vi "GUI_Bella_Control_Center_Staging.vi"() -> ()   [LabVIEW 2020]
uses:
  Shared/GUI_Template/GUI_master/tcp_new_data_event.ctl
  Shared/GUI_Template/GUI_master/tcp new data cluster.ctl
  GUI_TestStand/Fire button.ctl
  Device Drivers/DG645/subVIs/TriggerSource_TypDef.ctl
  delay scan start and end.ctl
  <vilib>/Utility/config.llb/Write Key (I32).vi
  <vilib>/Platform/browser.llb/Open URL in Default Browser (string).vi
  <vilib>/Utility/config.llb/NI_LVConfig.lvlib
panel:
  in  "GUIdevice 33":string="FLIP-1BL-Tel4FoilND1"
  in  "Position::33":enum16{"Unknown", "Position1", "Position2"}(ring) caption="1BLTel4Foil"
  in  "Uniblitz":bool=TRUE
  in  "value13::42":dbl=0.006 caption="Jet SC ChF PostScan" min=-9999999.0 max=9999999.0 format="%#_3f"
  in  "value12::42":dbl=0.006 caption="Jet  SC ChF Scan" min=-9999999.0 max=9999999.0 format="%#_3f"
  in  "GUIdevice 42":string="MANPAR-BELLA-OFI"
  in  "value15::42":dbl=0.006 caption="SC ChA PostScan" min=-9999999.0 max=9999999.0 format="%#_3f"
  in  "value14::42":dbl=0.006 caption="SC ChA Scan" min=-9999999.0 max=9999999.0 format="%#_3f"
  out "density down (10^18/cc)":dbl
  out "density up (10^18/cc)":dbl
  in  "Amplitude.Ch AB::13":dbl caption="Cap Trigger (V)" min=0.5 max=5.0 format="%.3p"
  in  "Delay.Ch A::13":dbl caption="Discharge delay A" min=-0.9 max=0.9 format="%.3p"
  in  "GUIdevice 13":string="DDG-AA-SRS2"
  in  "pressure::29":dbl caption="Dopant P set (Torr)" min=0.0 max=500.0 format="%.2f"
  out "pressure2::19":dbl caption="Pressure act DS (Torr)" min=-100.0 max=500.0 format="%.2f"
  out "pressure::19":dbl caption="Stage1 P act US (Torr)" min=-100.0 max=500.0 format="%.2f"
  in  "Delay.Ch B::13":dbl caption="Cap Trigger width" min=0.0 max=1e-05 step=1e-05 format="%.3p"
  in  "pressure::26":dbl caption="APL Pressure (Torr)" min=0.0 max=50.0 format="%.2f"
  out "Data.Channel 2::14":dbl caption="Flow US (sccm)" min=0.0 max=1000.0 format="%.1f"
  in  "Data.Channel 2::11":dbl caption="Stage1 P set US (Torr)" min=0.0 max=1000.0 format="%.2f"
  in  "SlaveValue::11":dbl caption="Slave Value (%)" min=0.0 max=1000.0 format="%.1f"
  out "Data.Channel 1::14":dbl caption="Flow DS (sccm)" min=0.0 max=1000.0 format="%.1f"
  in  "Data.Channel 1::11":dbl caption="Stage1 P set DS (Torr)" min=0.0 max=1000.0 format="%.2f"
  in  "GUIdevice 19":string="GAUGE-PL1-CapPressure"
  in  "Position.Ch3::18":dbl caption="stage 2 longitudinal" min=0.0 max=78.0
  in  "Position.Ch2::18":dbl caption="Stage 2 transverse" min=-100.0 max=100.0
  in  "Position.Ch4::18":dbl caption="Stage 2 vertical" min=0.0 max=40.0
  in  "GUIdevice 18":string="STAGE-PL1-Zaber"
  in  "position::16":dbl caption="tape vertical (mm)" min=-48.0 max=0.0
  in  "hex pos for SMF focal scan":dbl=6.5 caption="hex pos for SMF focus" format="%#_13g"
  in  "dist SMF to cap entrance":dbl=6.5 caption="dist SMF to cap entrance\n+ve SMF upstream" format="%#_13g"
  in  "value11::42":dbl caption="SMF focus on HPD" min=-9999999.0 max=9999999.0
  out "Focus into cap":dbl
  in  "GUIdevice 16":string="STAGE-PL1-Vertical"
  in  "wangle::30":dbl caption="w" min=-10.0 max=10.0 step=0.01 format="%.5f"
  in  "vangle::30":dbl caption="v" min=-5.0 max=5.0 step=0.01 format="%.5f"
  in  "uangle::30":dbl caption="u" min=-5.0 max=5.0 step=0.01 format="%.5f"
  in  "ypos::30":dbl caption="y" min=-10.0 max=10.0 step=0.01 format="%.5f"
  in  "zpos::30":dbl caption="z" min=-10.0 max=10.0 step=0.01 format="%.5f"
  in  "xpos::30":dbl caption="x" min=-25.0 max=25.0 step=0.01 format="%.5f"
  in  "GUIdevice 30":string="HEX-PL1-3"
  in  "GUIdevice 29":string="PRC-PL1-Stage1-Dopant"
  in  "Position.Ch1::44":dbl caption="Current Position" min=0.0 max=150.0 format="%.3f"
  in  "Position.Channel 2::31":T1(ring) caption="Little Rick"
  in  "GUIdevice 27":string="DDG-AA-SRS3"
  in  "GUIdevice 26":string="PRC-PL1-PressureAPL"
  in  "GUIdevice 20":string="HV-PL1-Glassman"
  in  "GUIdevice 14":string="GAUGE-PL1-FlowStage1"
  in  "GUIdevice 11":string="PRC-PL1-Stage1"
  in  "amplitude.Channel_A::27":dbl caption="Caps Trig (V) c unpl?" min=-3.0 max=4.0 format="%.2f"
  in  "voltage::20":dbl caption="Discharge HV (kV)" min=0.0 max=40.0 format="%.2f"
  in  "Delay.Ch B::10":dbl=-1.631e-06 caption="UniblitzOpenTime B\n(0 closed, 0.07 default)" min=-0.1 max=15.0 format="%.4f"
  in  "value6::42":dbl=0.006 caption="PostScanRate ChF" min=0.1 max=1.0 format="%#_3f"
  in  "value1::43":bool=TRUE caption="GasJetOn"
  in  "value0::43":bool=TRUE caption="SCS"
  in  "Delay.Ch H::32":dbl caption="Time width H" min=-0.1 max=0.01 format="%.3p"
  in  "Delay.Ch G::32":dbl caption="jet open G" min=-0.1 max=0.1 format="%.3p"
  in  "Delay.Ch D::32":dbl caption="Time Width D" min=-0.1 max=0.01 format="%.3p"
  in  "Delay.Ch E::32":dbl caption="jet open E" min=-0.1 max=0.03 format="%.3p"
  in  "Delay.Ch F::32":dbl caption="Time width F" min=-0.1 max=0.01 format="%.3p"
  in  "Delay.Ch C::32":dbl caption="jet open C" min=-0.1 max=0.1 format="%.3p"
  out "got manpar ofi bool data":bool
  out "got manpar ofi data":bool
  out "set expt editor":bool
  in  "Delay.Ch F::10":dbl=-1.631e-06 caption="Delay F" min=-0.1 max=10.0 format="%.4f"
  in  "Amplitude.Ch GH::10":dbl=-1.631e-06 caption="Shot Shutter V" min=0.5 max=5.0 format="%.1f"
  in  "Rate (Hz)":dbl=0.3
  in  "Allow Fire Continues":bool
  out "Fire continues Indicator":bool caption="firing"
  in  "Fire Button":T2=TRUE
  in  "Trigger.Source::10":T3 caption="SRS Trigger Mode"
  in  "value5::42":dbl=0.006 caption="1BL-2BL-\nSplitter-Rpcnt" min=-9999999.0 max=9999999.0 format="%#_6p"
  in  "value6::43":bool=TRUE caption="GhostFoil-In"
  in  "value5::43":bool=TRUE caption="1BL-Energy\nMeter-In"
  in  "value4::43":bool=TRUE caption="2BLFoil-In"
  in  "value3::43":bool=TRUE caption="1BLFoil-In"
  in  "value2::43":bool=TRUE caption="ClunkerIn"
  out "CurrentStatus":string
  in  "MoveStage":bool
  in  "GUIdevice 44":string="STAGE-LT-Megattenuator"
  in  "GUIdevice 43":string="MANPAR-BELLA-OFI-Boolean"
  in  "Pressure.device 2::39":dbl caption="Dopant pressure\nLow1down" min=-20.0 max=500.0 format="%.3f"
  out "HPD2 to match HPD":dbl
  out "HPD - focus":dbl
  in  "value1::42":dbl=230.0 caption="1BL focus pos" min=-9999999.0 max=9999999.0
  in  "position::23":dbl caption="position HPD2" min=0.0 max=600.0 format="%.1f"
  in  "position::3":dbl caption="position HPD" min=0.0 max=600.0 format="%.1f"
  in  "Save \ncreenshots":bool
  out "error out":errorcluster
  out "Hpd pos for jet exit":dbl
  in  "value2::42":dbl=276.0 caption="jet exit on hpd for hexX=0" min=-9999999.0 max=9999999.0
  in  "GUIdevice 41":string="STAGE-PL1-JetLength"
  in  "position::41":dbl caption="Jet Length pos" min=0.0 max=50.0 format="%.1f"
  out "lp mode HPDplane\n - HPD ref pos":dbl
  out "height above jet":dbl
  in  "value3::42":dbl=2.6 caption="zpos for 0 above jet" min=-9999999.0 max=9999999.0
  out "1BL delay (ns)\n+ is 1BL after 2BL":dbl
  in  "Position.Axis 1::8":dbl caption="1BL delay (mm)" min=-500.0 max=500.0 format="%.1f"
  in  "GUIdevice 8":string="STAGE-LT-1BLDelay"
  in  "Position.Channel 5::25":dbl caption="SMFiber (45in, 1out)" min=-60.0 max=55.0 format="%.1f"
  in  "Thales.DIAG_CU_Output_Percent_1::37":dbl caption="Amp2 att (%)" min=1.0 max=100.0 step=500.0 format="%.2f"
  in  "GUIdevice 37":string="SVE-LT-Thales"
  in  "Pressure.device 1::39":dbl caption="Hydrogen pressure\nHigh500" min=15.0 max=500.0 format="%.3f"
  in  "GUIdevice 39":string="PRC-PL1-HighPressure"
  in  "Scan":T4(ring)
  in  "LogTable":bool
  in  "New Google\nExpLog for new day?":bool=TRUE
  out "standard output":string
  in  "Create Log":bool caption="LogTable"
  in  "GUIdevice 38":string="STAGE-2BL-Compressor"
  in  "Position.Axis 1::38":dbl caption="Comp2 Translation" min=0.0 max=20.0 format="%.3f"
  in  "Position.Channel 5::31":T1(ring) caption="FROG foil"
  in  "AnalogOutput.Channel 1::36":dbl caption="M4A att (V)" min=0.0 max=5.0 step=500.0 format="%.2f"
  in  "GUIdevice 36":string="ATT-2BL-M4A"
  in  "GUIdevice 35":string="ATT-2BL-DM"
  in  "AnalogOutput.Channel 1::35":dbl caption="2BL DM att (V)" min=0.0 max=5.0 step=500.0 format="%.2f"
  in  "Delay.Ch B::32":dbl caption="Time width B" min=-0.1 max=0.01 format="%.3p"
  in  "Delay.Ch A::32":dbl caption="jet open A" min=-0.1 max=0.1 format="%.3p"
  in  "GUIdevice 32":string="DDG-AA-SRSGasJet-645"
  in  "position::6":dbl caption="LPmode stage long (605 safe)" min=0.0 max=50.0 format="%.1f"
  in  "GUIdevice 6":string="STAGE-PL1-LPmodeLong"
  in  "EnableMotor::6":bool caption="LPmode motor \nstatus"
  in  "GUIdevice 4":string="STAGE-PL1-Capstage1"
  in  "GUIdevice 31":string="FLIP-AA-1Wire"
  out "Crystal2":enum16{"In", "Out", "Unknown"}(ring)
  in  "wangle::28":dbl caption="w" min=-2.0 max=2.0 step=0.01 format="%.5f"
  in  "vangle::28":dbl caption="v" min=-5.0 max=5.0 step=0.01 format="%.5f"
  in  "uangle::28":dbl caption="u" min=-1.0 max=1.0 step=0.01 format="%.5f"
  in  "ypos::28":dbl caption="y" min=-3.0 max=3.0 step=0.01 format="%.5f"
  in  "zpos::28":dbl caption="z" min=-12.5 max=12.5 step=0.01 format="%.5f"
  in  "xpos::28":dbl caption="x" min=-10.0 max=15.0 step=0.01 format="%.5f"
  in  "GUIdevice 28":string="HEX-PL1-2"
  in  "Position.Channel 1::25":dbl caption="LPmode kicker (~1in, 75out)" min=-75.0 max=79.0 format="%.1f"
  in  "GUIdevice 25":string="STAGE-PL1-Smaract"
  in  "Heater Alignment Directions":bool
  in  "Position.Axis 3::15":dbl caption="XY" min=-3.0 max=16.0 format="%.4f"
  in  "Position.Axis 2::15":dbl caption="Y" min=-3.0 max=17.0 format="%.4f"
  in  "Position.Axis 1::15":dbl caption="X" min=-3.0 max=13.0 format="%.4f"
  in  "GUIdevice 24":string="STAGE-HEAT-TL1"
  in  "GUIdevice 23":string="STAGE-HPD-Far"
  in  "GUIdevice 22":string="MANPAR-BELLA-FireCont"
  out "Absolute discharge timing":dbl caption="delay from pk" format="%#.3p"
  in  "value0::22":bool caption="Fire continuosly"
  in  "GUIdevice 15":string="MCD-HEAT-ESP1"
  in  "GUIdevice 17":string="DDG-AA-SRS0"
  out "error IO 2":errorcluster
  out "fire::10":string
  out "tcp data event":T5
  in  "UDP error message":string
  in  "GUIdevice 2":string="MANPAR-BELLA-General"
  in  "GUIdevice 10":string="DDG-AA-ShotCntrl"
  in  "GUIdevice 1":string="HEX-PL1-1"
  in  "GUIdevice 3":string="STAGE-HPD-Tel"
  in  "<command>::1":bool caption="ABORT\nHEXAPOD"
  in  "Step size":dbl min=-22.0 max=22.0 format="%.5f"
  in  "wangle::1":dbl caption="w (F11 F12)" min=-6.0 max=6.0 step=0.01 format="%.5f"
  in  "vangle::1":dbl caption="v (F9 F10)" min=-6.0 max=1.0 step=0.01 format="%.5f"
  in  "uangle::1":dbl caption="u (F7 F8)" min=-6.0 max=6.0 step=0.01 format="%.5f"
  in  "ypos::1":dbl caption="y (F3 F4)" min=-8.0 max=8.0 step=0.01 format="%.5f"
  in  "zpos::1":dbl caption="z (PgU PgD)" min=-12.0 max=15.0 step=0.01 format="%.5f"
  in  "xpos::1":dbl caption="x (F1 F2)" min=-25.0 max=25.0 step=0.01 format="%.5f"
  in  "Position.Axis 1::9":dbl caption="Comp1 Translation" min=-50.0 max=50.0 format="%.3f"
  in  "GUIdevice 9":string="STAGE-1BL-Compression"
  in  "stop":bool
  # "Jet"
  # "BELLA CONTROL CENTER"
  # "Manual Pars"
  # "Scan"
  # "CAP"
  # "Tape Hex (sm)"
  # "1wire"
  # "needs manpar-bella-ofi on\nMANPAR-BELLA-OFI-Boolean"
  # "Discharge timing (s)"
  # "off overrides \nto 0 ->"
  # "Heater timing (s)"
  # "Attenuate"
  # "Megattenuator Stage"
  # "IN"
  # "OUT"
  # "HEX 2 APL"
  # "DG"
  # "Compressors"
  # "AB Uniblitz\nCD AND gate SRS2\nEF trigs SRS4 (jet)\nGH big SCS"
  # "Note: APL actually R660um and L 13cm"
  # "pos1=in"
  # "Heater Alignment"
  # "Heat ESP0"
  # "Heat ESP1"
  # "Heat Pico"
  # "HPD Stage"
  # "HEX 1 cap"
  # "\"+x\" is laser propagation direction"
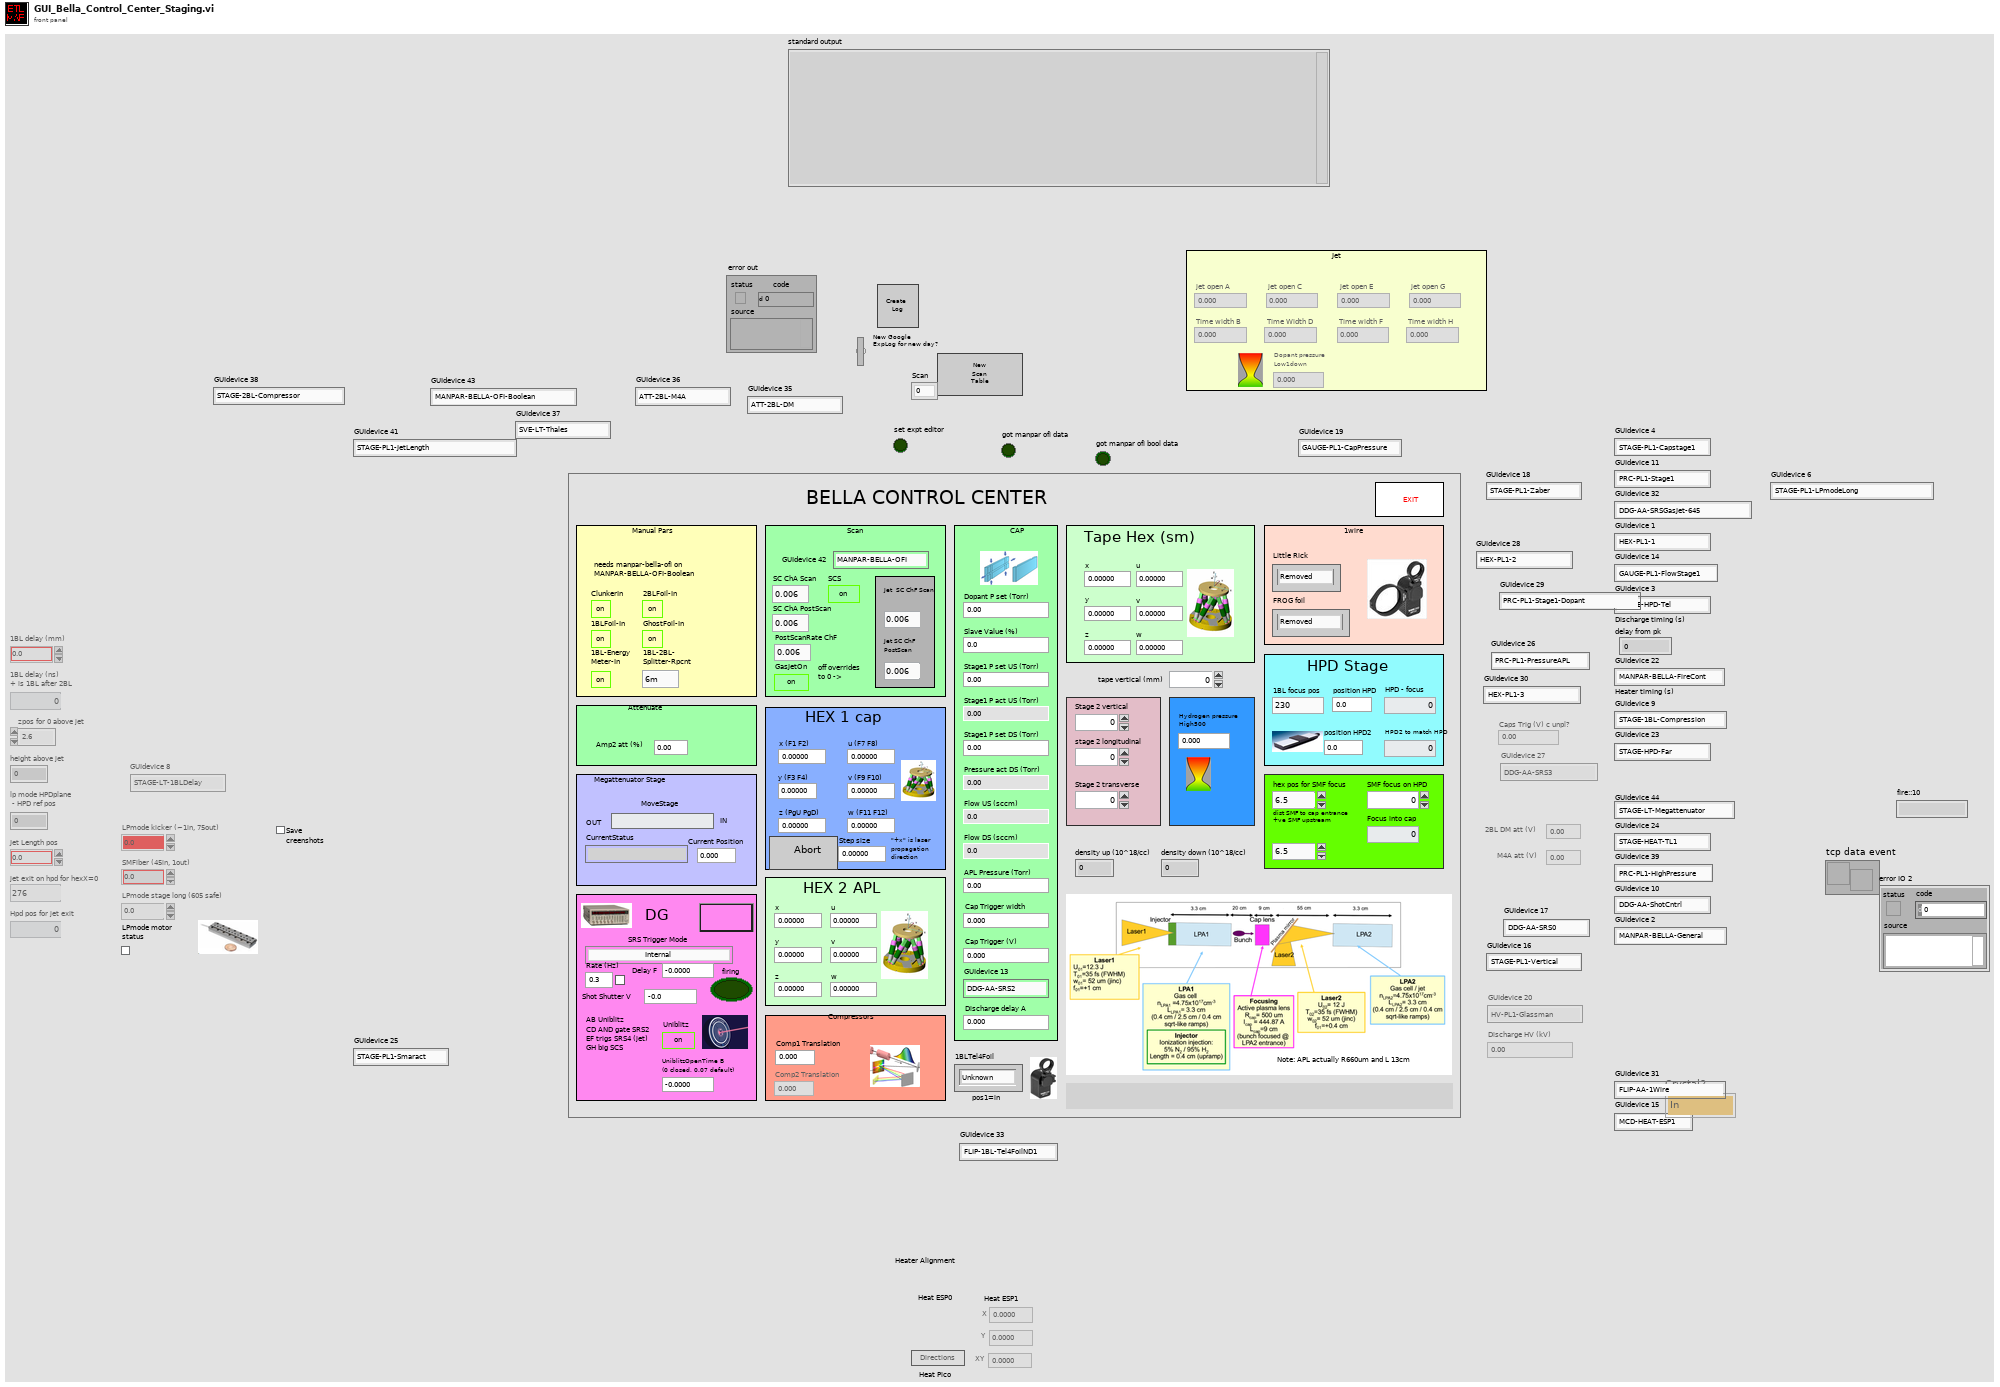
[diagram p1: front panel]
types:
  T1 = enum16{"Removed", "Inserted", "Unknown", "Moving"}
  T2 = typedef "Fire button.ctl" = bool
  T3 = typedef "TriggerSource_TypDef.ctl" = enum16{"Internal", "External rising edges", "External falling edges", "Single shot external rising edges", "Single shot external falling edges", "Single shot", "Line"}
  T4 = enum16{"0", "1", "2", "3", "4", "5", "6", "7", "8", "9", "10", "11", "12", "13", "14", "15", "16", "17", "18", "19", "20", "21", "22", "23", "24", "25", "26", "27", "28", "29", "30", "31", "32", "33", "34", "35", "36", "37", "38", "39", "40", "41", "42", "43", "44", "45", "46", "47", "48", "49", "50", "51", "52", "53", "54", "55", "56", "57", "58", "59", "60", "61", "62", "63", "64", "65", "66", "67", "68", "69", "70", "71", "72", "73", "74", "75", "76", "77", "78", "79", "81", "82", "83", "84", "85", "86", "87", "88", "89", "90", "91", "92", "93", "94", "95", "96", "97", "98", "99", ""}
  T5 = typedef "tcp_new_data_event.ctl" = refnum<user-event>
  T6 = typedef "tcp new data cluster.ctl" = cluster{"EventEnum":enum16{"new data", "connection status update"}, "Device name":string}
  T7 = enum8{"Enabled", "Disabled", "Disabled and Grayed Out"}
  T8 = enum32{"invalid app kind", "Development System", "Run Time System", "Student Edition", "Embedded LabVIEW", "Evaluation", "Custom"}
  T9 = enum32{"Invalid", "Standard", "Closed", "Hidden", "Minimized", "Maximized"}
  T10 = typedef "delay scan start and end.ctl" = cluster{"Channel":string, "Scan Start":dbl, "Scan End":dbl}
  T11 = typedef "imagedata.ctl" = cluster{"image type":i32, "image depth":i32, "image":u8[], "mask":u8[], "colors":u32[], "Rectangle":cluster{"left":i16, "top":i16, "right":i16, "bottom":i16}}
  T12 = typedef "NI_LVConfig.lvlib/Config Data RefNum.ctl" = refnum<k1>
  T13 = cluster{"Core":cluster{"Current VI Reference":refnum<vi>, "Close Panel on Exit?":bool}, "Heater timing offset":dbl, "Discharge timing offset":dbl, "Jet trigger":bool, "Tik1":u32, "Tik2":u32, "Fire Continues Allowed":bool}
  T14 = cluster{"Current VI Reference":refnum<vi>, "Close Panel on Exit?":bool}
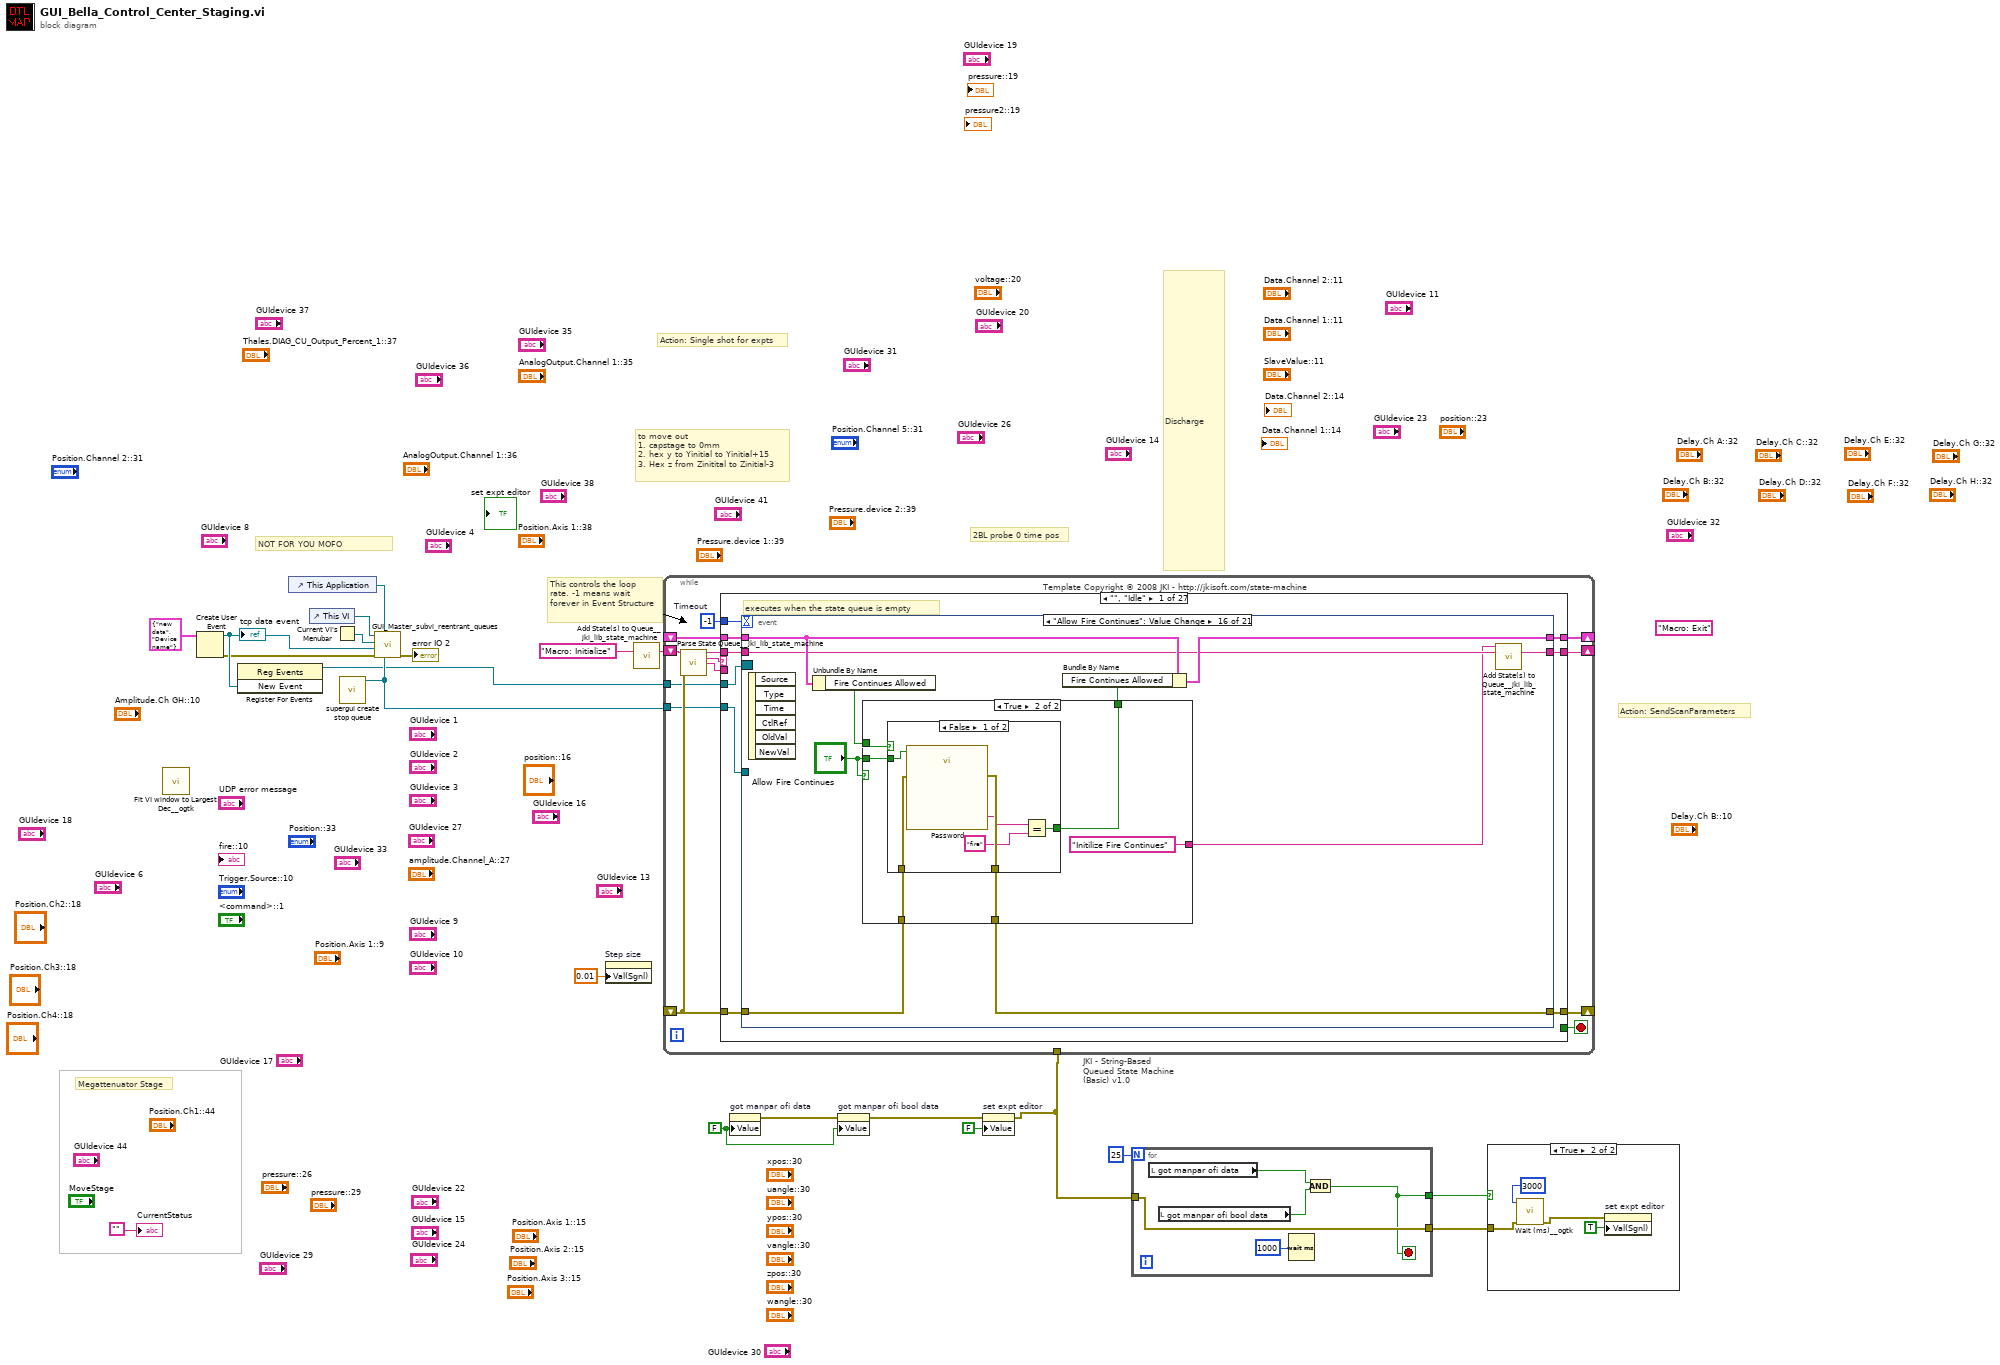
[diagram p0: block diagram]
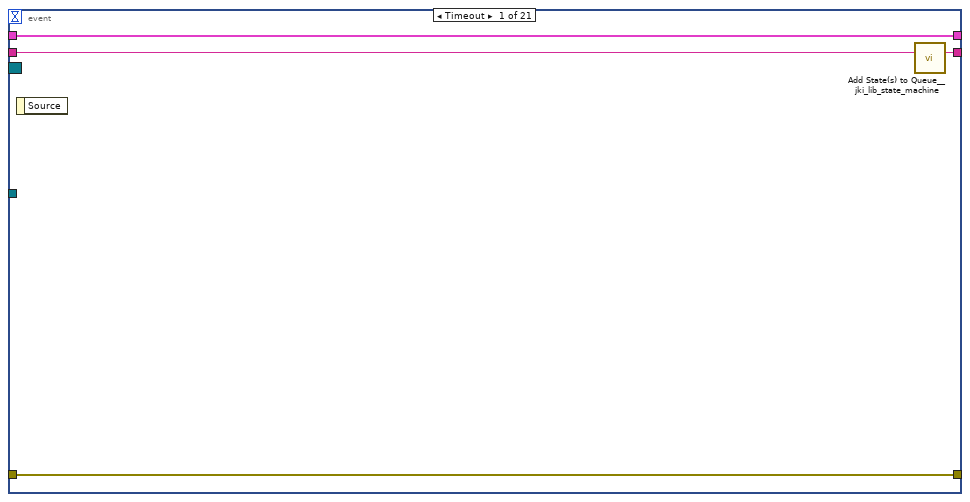
[diagram p3: hidden frame]
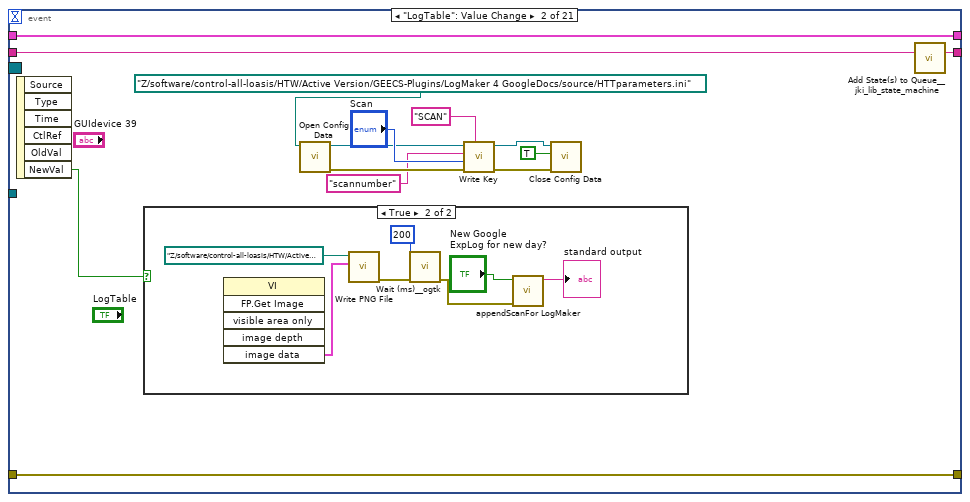
[diagram p4: hidden frame]
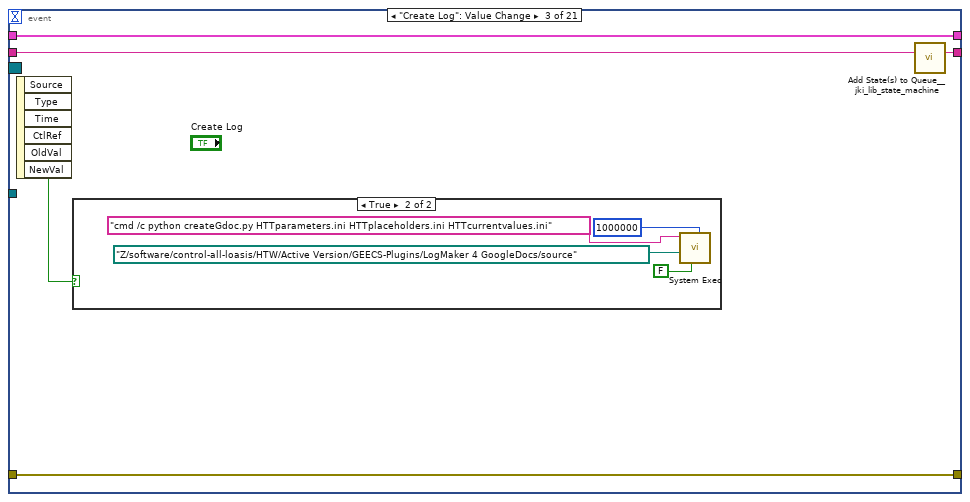
[diagram p6: hidden frame]
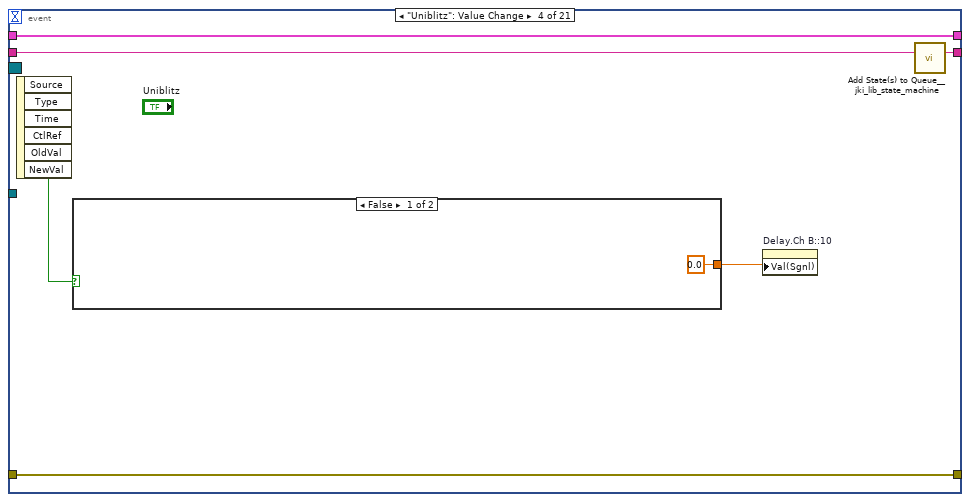
[diagram p8: hidden frame]
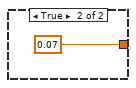
[diagram p9: hidden frame]
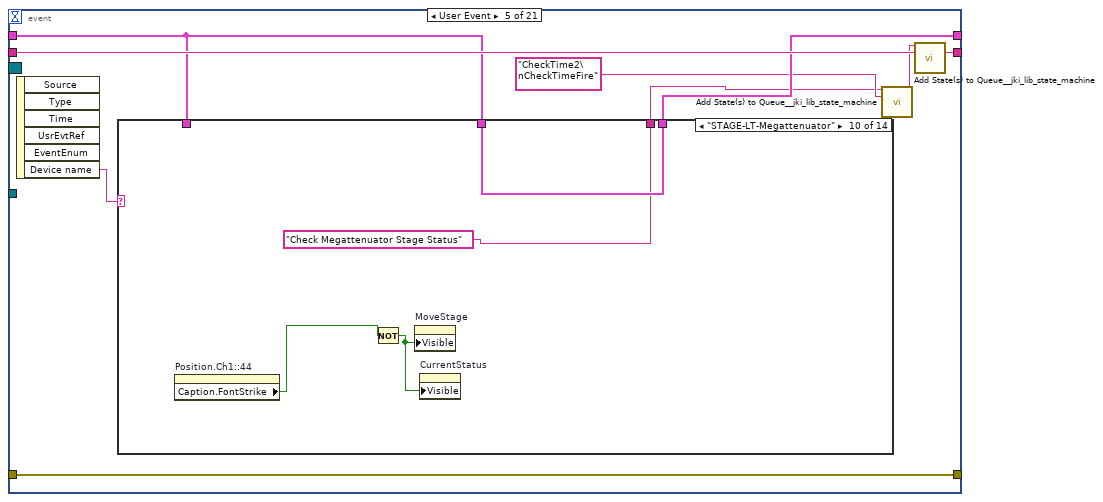
[diagram p10: hidden frame]
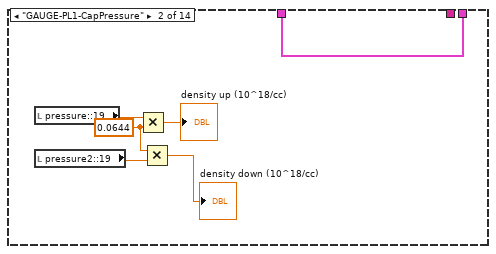
[diagram p12: hidden frame]
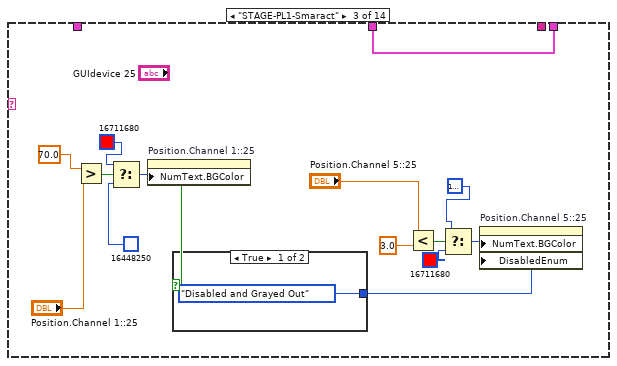
[diagram p13: hidden frame]
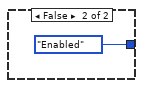
[diagram p14: hidden frame]
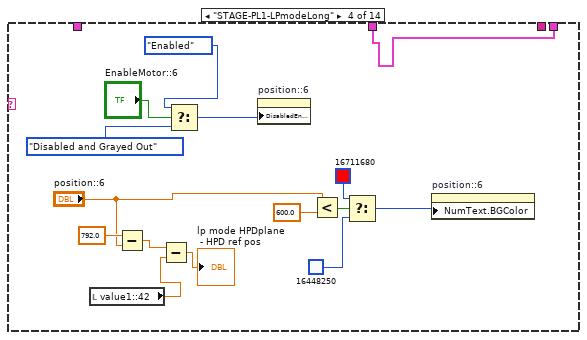
[diagram p15: hidden frame]
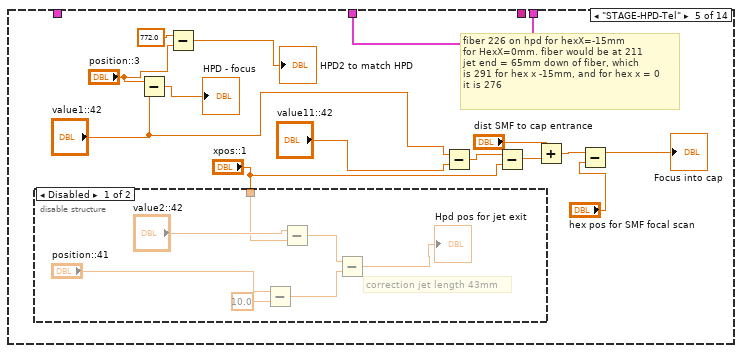
[diagram p16: hidden frame]
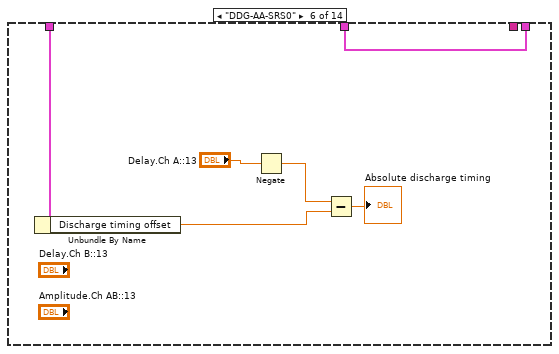
[diagram p18: hidden frame]
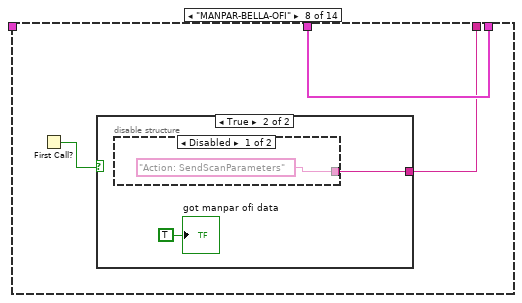
[diagram p20: hidden frame]
diagram:
  w5 = FALSE ("got manpar ofi data")
  (unwired) "Macro: Exit"
  # "Action: SendScanParameters"
  # "Discharge"
  # "Megattenuator Stage"
  # "2BL probe 0 time pos"
  # "Action: Single shot for expts"
  # "to move out\n1. capstage to 0mm\n2. hex y to Yinitial to Yinitial+15\n3. Hex z from Zinitital to Zinitial-3"
  # "This controls the loop rate. -1 means wait forever in Event Structure"
  # "NOT FOR YOU MOFO"
  n1 = call <userlib>:"Fit VI window to Largest Dec__ogtk.vi"() -> ()  [unwired: 6 in, 2 out]
  n2 = Create User Event(user event datatype=T6 {"EventEnum"=enum."new data", "Device name"="Device name"} ("New Event")) -> (user event=w20:refnum<user-event>, error out=w19:errorcluster)  [unwired: 1 in]
  "tcp data event" <- w20
  n3 = register-events(w20) -> (reference out=w10:refnum<event-registration>)  [unwired: 2 in, 1 out]
  n4 = control-ref of="This Application"() -> (w21:refnum<vi>)
  n5 = control-ref of="This VI"() -> (w14:refnum<vi>)
  n6 = Current VI's Menubar() -> (w17:refnum<k9>)
  n7 = call "supergui create stop queue.vi"() -> ("STOP Queue out"=w11:refnum<queue>)  [unwired: 11 in]
  n8 = call "GUI_Master_subvi_reentrant_queues.vi"("STOP Queue in"=w11, "This Application"=w21, "error in (no error)"=w19, "tcp data event"=w20, "Caller menu reference"=w17, "Caller VI ref"=w14) -> ("error out"=→"error IO 2":errorcluster)  [unwired: 5 in]
  n9 = property on="Step size" class="DigNum (strict)"("Val(Sgnl)"=0.01 ("Value (Signaling)")) -> ()  [unwired: 2 in, 2 out]
  n10 = call <vilib>:"Add State(s) to Queue__jki_lib_state_machine.vi"("State(s) in (\"\")"="Macro: Initialize") -> ("States Out"=w12:string)  [unwired: 14 in]
  n11 = property on="got manpar ofi data" class="Bool (strict)"("Value"=w5) -> (error out=w6:errorcluster)  [unwired: 2 in, 1 out]
  n12 = property on="got manpar ofi bool data" class="Bool (strict)"(error in=w6, "Value"=w5) -> (error out=w7:errorcluster)  [unwired: 1 in, 1 out]
  n13 = property on="set expt editor" class="Bool (strict)"(error in=w7, "Value"=FALSE ("set expt editor")) -> (error out=w4:errorcluster)  [unwired: 1 in, 1 out]
  n14 = while "JKI - String-Based Queued State Machine (Basic) v1.0" {
    shift-right: [w27] -> _
    shift-left: _ -> [w26]
    shift-right: [w30] -> _
    shift-left: _ -> [w24]
    shift-right: [w29] -> _
    shift-left: w12 -> [w31]
    tunnel: w10 -> [w23]
    tunnel: w11 -> [w22]
    tunnel: w4 -> [_]
    stop <- w28 stop-if-true
    w25 = -1  # Timeout
    # "Template Copyright © 2008 JKI - http://jkisoft.com/state-machine"
    n15 = call <vilib>:"Parse State Queue__jki_lib_state_machine.vi"("State Queue"=w31, "Error In (no error)"=w24) -> ("Remaining States"=w33:string, "Current State"=w34:string, "Arguments"=w32:string)  [unwired: 11 in]
    n16 = case shown="\"\", \"Idle\"" w34 {
      selector: w34 -> [_ _ w372 _ _ _ _ _ _ _ _ _ _ _ _ _ _ _ _ _ _ _ _ _ _ _ _]
      tunnel: w33 -> [w43 w371 w376 w394 w400 w405 w409 w420 w426 w430 w434 w440 w451 w477 w482 w495 w499 w505 w514 w551 w562 w574 w586 w595 w599 w634 w649]
      tunnel: w32 -> [_ _ _ _ _ _ _ _ _ _ _ w435 w445 _ _ _ _ _ _ _ _ _ _ _ _ _ _]
      tunnel: w26 -> [w41 w368 w374 w385 w397 w403 w406 _ w421 w427 w432 w438 w447 w474 w479 w492 w496 w502 w511 w539 w558 w568 w583 w593 w596 w631 w646]
      tunnel: [w40 w369 w378 w391 errorcluster {"status"=FALSE, "code"=0, "source"=""} ("error out") w402 w407 w417 w422 w428 w431 w436 w448 w475 w480 w493 w497 w503 w512 w549 w556 w563 w584 w590 w597 w632 w647] -> w30
      tunnel: w24 -> [w39 w369 w377 w391 w396 w402 w407 w417 w423 w428 w431 w437 w449 w475 w480 w493 w497 w503 w512 w549 w560 w564 w584 w591 w597 w632 w647]
      tunnel: [w42 w370 w375 w393 w399 w404 w408 w419 w425 w429 w433 w439 w450 w476 w481 w494 w498 w504 w513 w550 w561 w573 w585 w594 w598 w633 w648] -> w29
      tunnel: [_ _ _ _ _ TRUE _ _ _ _ _ _ _ _ _ _ _ _ _ _ _ _ _ _ _ _ _] -> w28
      tunnel: [w35 w368 w374 w392 w397 w403 w406 w418 w421 w427 w432 w438 w447 w474 w479 w492 w496 w502 w511 w548 w558 w567 w582 w593 w596 w631 w646] -> w27
      tunnel: w25 -> [w38 _ _ _ _ _ _ _ _ _ _ _ _ _ _ _ _ _ _ _ _ _ _ _ _ _ _]
      tunnel: w23 -> [w37 _ _ _ _ _ _ _ _ _ _ _ _ _ _ _ _ _ _ _ _ _ _ _ _ _ _]
      tunnel: w22 -> [w36 _ _ _ _ _ _ _ _ _ _ _ _ _ _ w484 _ _ _ _ _ _ _ _ _ _ _]
      frame "", "Idle" {
        # "executes when the state queue is empty"
        n17 = event shown="[15] \"Allow Fire Continues\": Value Change" {
          selector: w37 -> [_ _ _ _ _ _ _ _ _ _ _ _ _ _ _ _ _ _ _ _ _]
          dyn-events: _ -> [_ _ _ _ _ _ _ _ _ _ _ _ _ _ _ _ _ _ _ _ _]
          timeout: w38 -> [_ _ _ _ _ _ _ _ _ _ _ _ _ _ _ _ _ _ _ _ _]
          tunnel: w43 -> [w47 w61 w73 w83 w94 w215 w217 w222 w232 w242 w252 w262 w272 w278 w296 w305 w328 w333 w339 w341 w367]
          tunnel: [w46 w60 w72 w82 w93 w214 w218 w223 w233 w243 w253 w263 w273 w279 w296 w304 w328 w331 w339 w340 w366] -> w42
          tunnel: w41 -> [w44 w58 w70 w80 w90 w212 w220 w225 w235 w245 w255 w265 w275 w281 w295 w307 w329 w335 w338 w348 w364]
          tunnel: [w45 w59 w71 w81 w92 w213 w219 w224 w234 w244 w254 w264 w274 w280 w293 w310 w327 w334 w337 w347 w365] -> w40
          tunnel: w39 -> [w45 w59 w71 w81 w92 w213 w219 w224 w234 w244 w254 w264 w274 w280 w294 w309 w327 w334 w337 w347 w365]
          tunnel: [w44 w58 w70 w80 w89 w212 w220 w225 w235 w245 w255 w265 w275 w281 w295 w308 w329 w335 w338 w348 w364] -> w35
          tunnel: w36 -> [_ _ _ _ _ _ _ _ _ _ _ _ _ _ _ _ _ _ _ _ _]
          event Timeout {
            n18 = event-data() -> ()  [unwired: 1 in, 1 out]
            n19 = call <vilib>:"Add State(s) to Queue__jki_lib_state_machine.vi"("State(s) in (\"\")"=w47) -> ("States Out"=w46:string)  [unwired: 14 in]
          }
          event "LogTable": Value Change {
            n20 = event-data() -> ("NewVal"=w48:bool)  [unwired: 1 in, 5 out]
            n21 = case shown="True" w48 {
              frame False {
              }
              frame True {
                n22 = invoke class="VI" method="FP.Get Image"() -> ("image data"=w68:T11)  [unwired: 6 in, 5 out]
                n23 = call <vilib>:"Write PNG File.vi"("image data"=w68, "path to PNG file"=path "Z:/software/control-all-loasis/HTW/Active Version/GEECS-Plugins/LogMaker 4 GoogleDocs/source/frontpanel.png" ("report file path")) -> ("error out"=w63:errorcluster)  [unwired: 8 in, 1 out]
                n24 = call <userlib>:"Wait (ms)__ogtk.vi"("error in (no error)"=w63, "milliseconds to wait"=u32 200 ("millisecond timer value")) -> ("error out"=w62:errorcluster)  [unwired: 8 in, 1 out]
                n25 = call "appendScanFor LogMaker.vi"("error in (no error)"=w62, "New Google\nExpLog for new day?"="New Google\nExpLog for new day?") -> ("standard output"=→"standard output":string)  [unwired: 9 in]
              }
            }
            n26 = call <vilib>:"Open Config Data.vi"("configuration file path"=path "Z:/software/control-all-loasis/HTW/Active Version/GEECS-Plugins/LogMaker 4 GoogleDocs/source/HTTparameters.ini") -> ("error out"=w55:errorcluster, "refnum"=w53:T12)  [unwired: 8 in, 1 out]
            n27 = call-poly <vilib>:"Write Key.vi"("section"="SCAN", "error in (no error)"=w55, "value"="Scan", "key"="scannumber", "refnum"=w53) -> ("error out"=w56:errorcluster, "refnum out"=w54:T12)  [unwired: 4 in, 1 out]
            n28 = call <vilib>:"Close Config Data.vi"("error in (no error)"=w56, "write file if changed (T)"=TRUE, "refnum"=w54) -> ()  [unwired: 7 in, 2 out]
            n29 = call <vilib>:"Add State(s) to Queue__jki_lib_state_machine.vi"("State(s) in (\"\")"=w61) -> ("States Out"=w60:string)  [unwired: 14 in]
          }
          event "Create Log": Value Change {
            n30 = event-data() -> ("NewVal"=w69:bool)  [unwired: 1 in, 5 out]
            n31 = case shown="True" w69 {
              frame False {
              }
              frame True {
                n32 = call <vilib>:"System Exec.vi"("expected output size  (4096)"=u32 1000000, "run minimized? (F)"=FALSE, "working directory"=path "Z:/software/control-all-loasis/HTW/Active Version/GEECS-Plugins/LogMaker 4 GoogleDocs/source", "command line"="cmd /c python createGdoc.py HTTparameters.ini HTTplaceholders.ini HTTcurrentvalues.ini") -> ()  [unwired: 4 in, 4 out]
              }
            }
            n33 = call <vilib>:"Add State(s) to Queue__jki_lib_state_machine.vi"("State(s) in (\"\")"=w73) -> ("States Out"=w72:string)  [unwired: 14 in]
          }
          event "Uniblitz": Value Change {
            n34 = event-data() -> ("NewVal"=w79:bool)  [unwired: 1 in, 5 out]
            n35 = case shown="False" w79 {
              tunnel: [0.0 ("Value (Signaling)") 0.07 ("Value (Signaling)")] -> w78
              frame False {
              }
              frame True {
              }
            }
            n36 = property on="Delay.Ch B::10" class="DigNum (strict)"("Val(Sgnl)"=w78) -> ()  [unwired: 2 in, 2 out]
            n37 = call <vilib>:"Add State(s) to Queue__jki_lib_state_machine.vi"("State(s) in (\"\")"=w83) -> ("States Out"=w82:string)  [unwired: 14 in]
          }
          event User Event {
            n38 = event-data() -> ("Device name"=w91:string)  [unwired: 1 in, 5 out]
            n39 = case shown="\"STAGE-LT-Megattenuator\"" w91 {
              tunnel: w90 -> [_ _ _ _ _ w156 _ _ _ _ _ _ _ _]
              tunnel: w90 -> [w95 w101 w115 w132 w146 w154 w160 w163 w169 w176 w177 w188 w189 w210]
              tunnel: [w95 w101 w115 w132 w146 w154 w160 w163 w169 w176 w177 w188 w189 w210] -> w89
              tunnel: [_ _ _ _ _ _ _ w162 w168 "Check Megattenuator Stage Status" ("State(s) in Front (\"\")") _ _ _ _] -> w86
              frame "False", Default {
              }
              frame "GAUGE-PL1-CapPressure" {
                w99 = 0.0644 ("y")
                n40 = local read "pressure::19"() -> (w100:dbl)
                n41 = local read "pressure2::19"() -> (w98:dbl)
                n42 = Multiply(x=w100, y=w99) -> (x*y=→"density up (10^18/cc)":dbl)
                n43 = Multiply(x=w99, y=w98) -> (x*y=→"density down (10^18/cc)":dbl)
              }
              frame "STAGE-PL1-Smaract" {
                n44 = Greater?(x=70.0 ("y"), y="Position.Channel 1::25") -> (0:w102:bool)
                n45 = Select(t=u32 16711680, s=w102, f=u32 16448250) -> (s? t:f=w112:u32)
                n46 = property on="Position.Channel 1::25" class="DigNum (strict)"("NumText.BGColor"=w112) -> ()  [unwired: 2 in, 2 out]
                n47 = case shown="True" w102 {
                  tunnel: [T7."Disabled and Grayed Out" ("Disabled") T7."Enabled" ("Disabled")] -> w103
                  frame True {
                  }
                  frame False {
                  }
                }
                n48 = Less?(x="Position.Channel 5::25", y=3.0) -> (x < y?=w108:bool)
                n49 = Select(t=u32 16777225, s=w108, f=u32 16711680) -> (s? t:f=w111:u32)
                n50 = property on="Position.Channel 5::25" class="DigNum (strict)"("NumText.BGColor"=w111, "DisabledEnum"=w103) -> ()  [unwired: 2 in, 2 out]
              }
              frame "STAGE-PL1-LPmodeLong" {
                n51 = local read "value1::42"() -> (w119:dbl)
                n52 = Subtract(x=792.0, y="position::6") -> (x-y=w120:dbl)
                n53 = Subtract(x=w120, y=w119) -> (x-y=→"lp mode HPDplane\n - HPD ref pos":dbl)
                n54 = Select(t=T7."Enabled" ("Disabled"), s="EnableMotor::6", f=T7."Disabled and Grayed Out" ("Disabled")) -> (s? t:f=w123:T7)
                n55 = property on="position::6" class="DigNum (strict)"("DisabledEnum"=w123) -> ()  [unwired: 2 in, 2 out]
                n56 = Less?(x="position::6", y=600.0) -> (x < y?=w131:bool)
                n57 = Select(t=u32 16711680, s=w131, f=u32 16448250) -> (s? t:f=w127:u32)
                n58 = property on="position::6" class="DigNum (strict)"("NumText.BGColor"=w127) -> ()  [unwired: 2 in, 2 out]
              }
              frame "STAGE-HPD-Tel" {
                # "fiber 226 on hpd for hexX=-15mm\nfor HexX=0mm. fiber would be at 211\njet end = 65mm down of fiber, which\nis 291 for hex x -15mm, and for hex x = 0\nit is 276"
                n59 = disable-structure shown="Disabled" {
                  disable-tunnel: "xpos::1" -> [w147 _]
                  frame Disabled {
                    # "correction jet length 43mm"
                    n60 = Subtract(x="position::41", y=10.0) -> (x-y=w149:dbl)
                    n61 = Subtract(x="value2::42", y=w147) -> (x-y=w150:dbl)
                    n62 = Subtract(x=w150, y=w149) -> (x-y=→"Hpd pos for jet exit":dbl)
                  }
                  frame Enabled {
                  }
                }
                n63 = Subtract(x="position::3", y="value1::42") -> (x-y=→"HPD - focus":dbl)
                n64 = Subtract(x=772.0 ("y"), y="position::3") -> (x-y=→"HPD2 to match HPD":dbl)
                n65 = Subtract(x="value1::42", y="value11::42") -> (x-y=w140:dbl)
                n66 = Subtract(x=w140, y="xpos::1") -> (x-y=w138:dbl)
                n67 = Add(x="dist SMF to cap entrance", y=w138) -> (x+y=w136:dbl)
                n68 = Subtract(x=w136, y="hex pos for SMF focal scan") -> (x-y=→"Focus into cap":dbl)
              }
              frame "DDG-AA-SRS0" {
                n69 = Unbundle By Name(w156) -> ("Discharge timing offset"=w155:dbl)
                n70 = Negate(x="Delay.Ch A::13") -> (-x=w157:dbl)
                n71 = Subtract(x=w157, y=w155) -> (x-y=→"Absolute discharge timing":dbl)
              }
              frame "STAGE-2BL-ProbeDelay" {
              }
              frame "MANPAR-BELLA-OFI" {
                n72 = First Call?() -> (First Call?: T/F=w161:bool)
                n73 = case shown="True" w161 {
                  tunnel: [_ w165] -> w162
                  frame False {
                  }
                  frame True {
                    n74 = disable-structure shown="Disabled" {
                      disable-tunnel: ["Action: SendScanParameters" ("State(s) in Front (\"\")") _] -> w165
                      frame Disabled {
                      }
                      frame Enabled {
                      }
                    }
                    "got manpar ofi data" <- TRUE ("got manpar ofi data")
                  }
                }
              }
              frame "MANPAR-BELLA-OFI-Boolean" {
                n75 = First Call?() -> (First Call?: T/F=w167:bool)
                n76 = case shown="True" w167 {
                  tunnel: [_ w171] -> w168
                  frame False {
                  }
                  frame True {
                    n77 = disable-structure shown="Disabled" {
                      disable-tunnel: ["Action: SendScanParameters" ("State(s) in Front (\"\")") _] -> w171
                      frame Disabled {
                      }
                      frame Enabled {
                      }
                    }
                    "got manpar ofi bool data" <- TRUE ("got manpar ofi bool data")
                  }
                }
              }
              frame "STAGE-LT-Megattenuator" {
                n78 = property on="Position.Ch1::44" class="DigNum (strict)"() -> ("Caption.FontStrike"=w173:bool)  [unwired: 2 in, 2 out]
                n79 = Not(x=w173) -> (.not. x?=w174:bool)
                n80 = property on="MoveStage" class="Bool (strict)"("Visible"=w174) -> ()  [unwired: 2 in, 2 out]
                n81 = property on="CurrentStatus" class="Str"("Visible"=w174) -> ()  [unwired: 2 in, 2 out]
              }
              frame "STAGE-LT-1BLDelay" {
                n82 = disable-structure shown="Disabled" {
                  frame Disabled {
                    n83 = Subtract(x="Position.Axis 1::8", y=929.0) -> (x-y=w186:dbl)
                    n84 = Negate(x=w186) -> (-x=w185:dbl)
                    n85 = Multiply(x=2.0, y=w185) -> (x*y=w183:dbl)
                    n86 = Divide(x=w183, y=299792458000.0) -> (x/y=w181:dbl)
                    n87 = Multiply(x=1000000000.0, y=w181) -> (x*y=→"1BL delay (ns)\n+ is 1BL after 2BL":dbl)
                  }
                  frame Enabled {
                  }
                }
              }
              frame "1WIRE-BELLA-Flipper" {
              }
              frame "HEX-PL1-2" {
                n88 = disable-structure shown="Disabled" {
                  frame Disabled {
                    n89 = disable-structure shown="Disabled" {
                      disable-tunnel: "ypos::28" -> [w194 _]
                      frame Disabled {
                        n90 = Equal?(x=w194, y=15.6) -> (x = y?=w192:bool)
                        n91 = Equal?(x=-20.0 ("y"), y=w194) -> (x = y?=w196:bool)
                        n92 = case shown="False" w196 {
                          tunnel: [w200 enum16{"In", "Out"}."Out" ("sdfsdfs 2")] -> w191
                          tunnel: [w198 u32 16185078] -> w195
                          tunnel: w192 -> [w199 _]
                          frame False {
                            n93 = case shown="False" w199 {
                              tunnel: [enum16{"In", "Out", "Unknown"}."Unknown" ("sdfsdfs 2") enum16{"In", "Out"}."In" ("sdfsdfs 2")] -> w200
                              tunnel: [u32 16761154 ("Color Box") u32 16711680] -> w198
                              frame False {
                              }
                              frame True {
                              }
                            }
                          }
                          frame True {
                          }
                        }
                        "Crystal2" <- w191
                        n94 = property on="Crystal2" class="Enum (strict)"("RingText.FG Color"=w195, "RingText.BGColor"=w195) -> ()  [unwired: 2 in, 2 out]
                      }
                      frame Enabled {
                      }
                    }
                  }
                  frame Enabled {
                  }
                }
              }
              frame "HEX-PL1-1" {
                n95 = Subtract(x="value3::42", y="zpos::1") -> (x-y=→"height above jet":dbl)
              }
            }
            n96 = call <vilib>:"Add State(s) to Queue__jki_lib_state_machine.vi"("State(s) in Front (\"\")"=w86, "State(s) in (\"\")"="CheckTime2\nCheckTimeFire" ("State(s) in Front (\"\")")) -> ("States Out"=w87:string)  [unwired: 13 in]
            n97 = call <vilib>:"Add State(s) to Queue__jki_lib_state_machine.vi"("State(s) in Front (\"\")"=w87, "State(s) in (\"\")"=w94) -> ("States Out"=w93:string)  [unwired: 13 in]
          }
          event "stop": Value Change {
            # "Exit Button Value Change (pressed) Event\n(this executes Macro: Exit to terminate the VI)"
            n98 = event-data() -> ()  [unwired: 1 in, 6 out]
            n99 = call <vilib>:"Add State(s) to Queue__jki_lib_state_machine.vi"("State(s) in Front (\"\")"="Macro: Exit", "State(s) in (\"\")"=w215) -> ("States Out"=w214:string)  [unwired: 13 in]
          }
          event Value Change {
            n100 = event-data() -> ()  [unwired: 1 in, 6 out]
            n101 = call <vilib>:"Add State(s) to Queue__jki_lib_state_machine.vi"("State(s) in Front (\"\")"="Action: Fire" ("State(s) in Front (\"\")"), "State(s) in (\"\")"=w217) -> ("States Out"=w218:string)  [unwired: 13 in]
          }
          event "value0::43", "value1::43", "value6::42", "value13::42", "value14::42", "value15::42": Value Change {
            n102 = event-data() -> ()  [unwired: 1 in, 6 out]
            n103 = call <vilib>:"Add State(s) to Queue__jki_lib_state_machine.vi"("State(s) in Front (\"\")"="Action: SendScanParameters" ("State(s) in Front (\"\")"), "State(s) in (\"\")"=w222) -> ("States Out"=w223:string)  [unwired: 13 in]
          }
          event "value2::43": Value Change {
            n104 = event-data() -> ()  [unwired: 1 in, 6 out]
            n105 = local read "GUIdevice 43"() -> (w226:string)
            n106 = Select(t="on", s="value2::43", f="off") -> (s? t:f=w231:string)
            n107 = call "DefaultValue_Variable_MC.vi"("Variable In"="value2", "Default Value"=w231, "Device In"=w226) -> ()  [unwired: 1 in]
            n108 = call <vilib>:"Add State(s) to Queue__jki_lib_state_machine.vi"("State(s) in (\"\")"=w232) -> ("States Out"=w233:string)  [unwired: 14 in]
          }
          event "value3::43": Value Change {
            n109 = event-data() -> ()  [unwired: 1 in, 6 out]
            n110 = local read "GUIdevice 43"() -> (w237:string)
            n111 = Select(t="on", s="value3::43", f="off") -> (s? t:f=w241:string)
            n112 = call "DefaultValue_Variable_MC.vi"("Variable In"="value3", "Default Value"=w241, "Device In"=w237) -> ()  [unwired: 1 in]
            n113 = call <vilib>:"Add State(s) to Queue__jki_lib_state_machine.vi"("State(s) in (\"\")"=w242) -> ("States Out"=w243:string)  [unwired: 14 in]
          }
          event "value4::43": Value Change {
            n114 = event-data() -> ()  [unwired: 1 in, 6 out]
            n115 = local read "GUIdevice 43"() -> (w247:string)
            n116 = Select(t="on", s="value4::43", f="off") -> (s? t:f=w251:string)
            n117 = call "DefaultValue_Variable_MC.vi"("Variable In"="value4", "Default Value"=w251, "Device In"=w247) -> ()  [unwired: 1 in]
            n118 = call <vilib>:"Add State(s) to Queue__jki_lib_state_machine.vi"("State(s) in (\"\")"=w252) -> ("States Out"=w253:string)  [unwired: 14 in]
          }
          event "value5::43": Value Change {
            n119 = event-data() -> ()  [unwired: 1 in, 6 out]
            n120 = local read "GUIdevice 43"() -> (w257:string)
            n121 = Select(t="on", s="value5::43", f="off") -> (s? t:f=w261:string)
            n122 = call "DefaultValue_Variable_MC.vi"("Variable In"="value5", "Default Value"=w261, "Device In"=w257) -> ()  [unwired: 1 in]
            n123 = call <vilib>:"Add State(s) to Queue__jki_lib_state_machine.vi"("State(s) in (\"\")"=w262) -> ("States Out"=w263:string)  [unwired: 14 in]
          }
          event "value6::43": Value Change {
            n124 = event-data() -> ()  [unwired: 1 in, 6 out]
            n125 = local read "GUIdevice 43"() -> (w267:string)
            n126 = Select(t="on", s="value6::43", f="off") -> (s? t:f=w271:string)
            n127 = call "DefaultValue_Variable_MC.vi"("Variable In"="value6", "Default Value"=w271, "Device In"=w267) -> ()  [unwired: 1 in]
            n128 = call <vilib>:"Add State(s) to Queue__jki_lib_state_machine.vi"("State(s) in (\"\")"=w272) -> ("States Out"=w273:string)  [unwired: 14 in]
          }
          event "value5::42", "value12::42": Value Change {
            n129 = event-data() -> ()  [unwired: 1 in, 6 out]
            n130 = flat-sequence {
              tunnel: ["GUIdevice 42"] -> w277
              tunnel: w277 -> [w288]
              frame #0 {
                n131 = Number To Fractional String(number="value5::42", precision (6)=i16 4) -> (F-format string=w283:string)  [unwired: 2 in]
                n132 = call "DefaultValue_Variable_MC.vi"("Variable In"="value5", "Default Value"=w283, "Device In"="GUIdevice 42") -> ()  [unwired: 1 in]
              }
              frame #1 {
                n133 = local read "value12::42"() -> (w287:dbl)
                n134 = Number To Fractional String(number=w287, precision (6)=i16 4) -> (F-format string=w291:string)  [unwired: 2 in]
                n135 = call "DefaultValue_Variable_MC.vi"("Variable In"="value5", "Default Value"=w291, "Device In"=w288) -> ()  [unwired: 1 in]
              }
            }
            n136 = call <vilib>:"Add State(s) to Queue__jki_lib_state_machine.vi"("State(s) in (\"\")"=w278, "State(s) at Back (\"\")"="Action: SendScanParameters" ("State(s) at Back (\"\")")) -> ("States Out"=w279:string)  [unwired: 13 in]
          }
          event "Heater Alignment Directions": Value Change {
            n137 = event-data() -> ()  [unwired: 1 in, 6 out]
            n138 = case shown="True" "Heater Alignment Directions" {
              tunnel: w294 -> [w297 w300]
              tunnel: [w297 w299] -> w293
              frame False {
              }
              frame True {
                n139 = call-poly <vilib>:"Open URL in Default Browser.vi"("error in (no error)"=w300, "URL"="https://docs.google.com/document/d/1RMZp6W8Kkog2nkTymSjyZ2bh9D7Vo4bxhvGgn3Ut4KE/edit") -> ("error out"=w299:errorcluster)  [unwired: 4 in, 1 out]
              }
            }
          }
          event "Allow Fire Continues": Value Change {
            n140 = event-data() -> ()  [unwired: 1 in, 6 out]
            n141 = Unbundle By Name(w307) -> ("Fire Continues Allowed"=w306:bool)
            n142 = case shown="True" "Allow Fire Continues" {
              tunnel: [w311 w318] -> w310
              tunnel: "Allow Fire Continues" -> [_ w317]
              tunnel: w309 -> [w311 w316]
              tunnel: w306 -> [w312 w315]
              tunnel: [w312 w313] -> w302
              tunnel: [_ "Initilize Fire Continues" ("State(s) in Front (\"\")")] -> w301
              frame False {
              }
              frame True {
                n143 = case shown="False" w315 {
                  tunnel: [w324 w325] -> w318
                  tunnel: w317 -> [w323 _]
                  tunnel: w316 -> [w322 w325]
                  tunnel: [w319 FALSE] -> w313
                  frame False {
                    n144 = call "Password"("Enable"=w323, "error in (no error)"=w322) -> ("Password"=w321:string, "error out"=w324:errorcluster)  [unwired: 15 in, 1 out]
                    n145 = Equal?(x=w321, y="fire") -> (x = y?=w319:bool)
                  }
                  frame True {
                  }
                }
              }
            }
            n146 = Bundle By Name(cluster=w307, "Fire Continues Allowed"=w302) -> (w308:T13)
            n147 = call <vilib>:"Add State(s) to Queue__jki_lib_state_machine.vi"("State(s) in Front (\"\")"=w301, "State(s) in (\"\")"=w305) -> ("States Out"=w304:string)  [unwired: 13 in]
          }
          event "Step size": Value Change {
            n148 = event-data() -> ("NewVal"=w330:dbl)  [unwired: 1 in, 5 out]
            n149 = property on="uangle::1" class="DigNum (strict)"("Increment"=w330) -> ()  [unwired: 2 in, 2 out]
            n150 = property on="vangle::1" class="DigNum (strict)"("Increment"=w330) -> ()  [unwired: 2 in, 2 out]
            n151 = property on="xpos::1" class="DigNum (strict)"("Increment"=w330) -> ()  [unwired: 2 in, 2 out]
            n152 = property on="zpos::1" class="DigNum (strict)"("Increment"=w330) -> ()  [unwired: 2 in, 2 out]
            n153 = property on="wangle::1" class="DigNum (strict)"("Increment"=w330) -> ()  [unwired: 2 in, 2 out]
            n154 = property on="ypos::1" class="DigNum (strict)"("Increment"=w330) -> ()  [unwired: 2 in, 2 out]
          }
          event "set expt editor": Value Change {
            n155 = event-data() -> ()  [unwired: 1 in, 6 out]
            n156 = call <vilib>:"Add State(s) to Queue__jki_lib_state_machine.vi"("State(s) in Front (\"\")"="Action: SendScanParameters" ("State(s) in Front (\"\")"), "State(s) in (\"\")"=w333) -> ("States Out"=w331:string)  [unwired: 13 in]
          }
          event Value Change {
            n157 = event-data() -> ()  [unwired: 1 in, 6 out]
            n158 = property on="value0::22" class="Bool (strict)"("Val(Sgnl)"=FALSE) -> ()  [unwired: 2 in, 2 out]
          }
          event "MoveStage": Value Change {
            n159 = event-data() -> ("OldVal"=w343:bool, "NewVal"=w346:bool)  [unwired: 1 in, 4 out]
            n160 = flat-sequence {
              tunnel: w346 -> [w353]
              tunnel: [w353] -> w345
              tunnel: [w350] -> w344
              tunnel: w343 -> [w349]
              tunnel: [w349] -> w342
              tunnel: w345 -> [w356]
              tunnel: w344 -> [w355]
              tunnel: w342 -> [w354]
              frame #0 {
                n161 = call "PasswordPrompt.vi"() -> ("Please enter password below 2"=w352:string)  [unwired: 11 in]
                n162 = Equal?(x=w352, y="l0dat&srv!") -> (x = y?=w350:bool)
              }
              frame #1 {
                n163 = case shown="False" w355 {
                  tunnel: w356 -> [_ w359]
                  tunnel: w354 -> [w357 _]
                  frame False {
                    n164 = property on="MoveStage" class="Bool (strict)"("Value"=w357) -> ()  [unwired: 2 in, 2 out]
                    n165 = call "Display Message to User"("Message"="Wrong Password") -> ()  [unwired: 9 in, 2 out]
                  }
                  frame True {
                    n166 = property on="MoveStage" class="Bool (strict)"("Value"=w359) -> ()  [unwired: 2 in, 2 out]
                    n167 = case shown="True" w359 {
                      frame False {
                        n168 = property on="Position.Ch1::44" class="DigNum (strict)"("Val(Sgnl)"=150.0 ("Value (Signaling)")) -> ()  [unwired: 2 in, 2 out]
                      }
                      frame True {
                        n169 = property on="Position.Ch1::44" class="DigNum (strict)"("Val(Sgnl)"=0.5 ("Value (Signaling)")) -> ()  [unwired: 2 in, 2 out]
                      }
                    }
                  }
                }
              }
            }
            n170 = call <vilib>:"Add State(s) to Queue__jki_lib_state_machine.vi"("State(s) in (\"\")"=w341) -> ("States Out"=w340:string)  [unwired: 14 in]
          }
          event Panel Close? {
            # "Discard the event because we'll close the front panel ourselves in Macro: Exit"
            # "Close Panel button (pressed) Event\n(this executes Macro: Exit to terminate the VI)"
            n171 = event-data() -> ()  [unwired: 1 in, 1 out]
            n172 = event-data("Discard?"=TRUE) -> ()  [unwired: 1 in, 1 out]
            n173 = call <vilib>:"Add State(s) to Queue__jki_lib_state_machine.vi"("State(s) in Front (\"\")"="Macro: Exit", "State(s) in (\"\")"=w367) -> ("States Out"=w366:string)  [unwired: 13 in]
          }
        }
      }
      frame "---------- Core ----------" {
        # "Do not put any code in this frame.\n(it is a separator no-op)"
        n174 = call <vilib>:"Add State(s) to Queue__jki_lib_state_machine.vi"("State(s) in (\"\")"=w371) -> ("States Out"=w370:string)  [unwired: 14 in]
      }
      frame Default {
        w381 = 42 items=["No error", "Argument error", "Memory is full", "Out of zone", "End of file", "File already open", "Generic file I/O error", "File not found", "File permission error", "Disk is full", "Duplicate path", "Too many files open", "System feature not enabled", "Resource file not found", "Cannot add resource", "Resource not found", "Image not found", "Image memory error", "Pen does not exist", "Config type invalid", "Config token not found", "Config parse error", "Config memory error", "Bad external code format", "Bad external code offset", "External code not present", "Null window", "Destroy window error", "Null menu", "Print aborted", "Bad print record", "Print driver error", "Windows error during printing", "Memory error during printing", "Print dialog error", "Generic print error", "Invalid device refnum", "Device not found", "Device parameter error", "Device unit error", "Cannot open device", "Device call aborted", "Generic error", "Cancelled by user", "Object ID too low", "Object ID too high", "Object not in heap", "Unknown heap", "Unknown object (invalid DefProc)", "Unknown object (DefProc not in table)", "Message out of range", "Invalid (null) method", "Unknown message", "Manager call not supported", "Bad address", "Network operation in progress", "Network operation timed out", "Connection is busy", "Network attribute not supported", "Network error", "Address in use", "System out of memory", "Connection aborted", "Connection refused", "Not connected", "Already connected", "Connection closed", "Initialization error (interapplication manager)", "Bad occurrence", "Wait on unbound occurrence handler", "Occurrence queue overflow", "Datalog type conflict", "Unused", "Unrecognized type (interapplication manager)", "Memory corrupt", "Failed to make temporary DLL", "Old CIN version", "Drag socket not found", "Failed to load drop-object", "Failed to register OLE object", "Failed to release OLE object", "Format specifier type mismatch", "Unknown format specifier", "Too few format specifiers", "Too many format specifiers", "Scan failed", "Newer CIN version", "Error converting to variant", "Runtime menu error", "Password tampered", "Variant attribute not found", "Incompatible variant data type", "Event data is not available", "Event Store is not present", "Occurrence is not found", "Event Queue is not created", "Event info is not available", "Refnum passed is NULL", "Error retrieving Class GUID", "Error retrieving CoClass GUID", "Error retrieving TypeLib GUID.", "Bad built application magic bytes.", "Specific driver is different from the specific driver associated with the Logical Name.", "There is no session opened to the class driver.", "Max Error", "MAX - Error with config objects", "MAX - Error loading configuration", "MAX - Group not supported"]
        # "Current State"
        # "Do not delete, rename, or modify this frame.\n(this is used to capture unhandled states and typos)"
        # "Handle mistyped state name (developer tool)"
        n175 = Format Into String(format string="Software Exception: Unhandled State \"%s\"." ("message"), error in=w377, w372) -> (resulting string=w380:string, error out=w379:errorcluster)  [unwired: 1 in]
        n176 = call <vilib>:"Error Cluster From Error Code.vi"("show call chain? (False)"=TRUE, "error in (no error)"=w379, "error message (\"\")"=w380, "error code (0)"=w381) -> ("error out"=w378:errorcluster)  [unwired: 5 in]
        n177 = call <vilib>:"Add State(s) to Queue__jki_lib_state_machine.vi"("State(s) in (\"\")"=w376) -> ("States Out"=w375:string)  [unwired: 14 in]
      }
      frame "Initialize Core Data" {
        # "Do not delete, rename, or modify this frame.\n(this is used to determine panel behavior on exit)"
        # "originally closed?"
        # "exe?"
        # "If panel starts closed or is an EXE, then close it when we exit"
        n178 = property class="VI"() -> ("Front Panel.Open"=w390:bool)  [unwired: 2 in, 2 out]
        n179 = property class="App"() -> ("App.Kind"=w389:T8)  [unwired: 2 in, 2 out]
        n180 = control-ref of="Current VI Reference"() -> (w383:refnum<vi>)
        n181 = Not(x=w390) -> (.not. x?=w387:bool)
        n182 = Equal?(x=w389, y=T8."Run Time System" ("Application:Kind")) -> (x = y?=w386:bool)
        n183 = Or(x=w387, y=w386) -> (x .or. y?=w384:bool)
        n184 = Bundle By Name(cluster=w385, "Core.Current VI Reference"=w383, "Core.Close Panel on Exit?"=w384) -> (w392:T13)
        n185 = call <vilib>:"Add State(s) to Queue__jki_lib_state_machine.vi"("State(s) in (\"\")"=w394) -> ("States Out"=w393:string)  [unwired: 14 in]
      }
      frame "Error Handler" {
        # "Unhandled Error -- Display it"
        # "Handle any errors here.\nYou can also output any states to clean-up after errors occur"
        # "Clear error"
        n186 = call <vilib>:"General Error Handler.vi"("error in (no error)"=w396) -> ()  [unwired: 10 in, 5 out]
        n187 = call <vilib>:"Add State(s) to Queue__jki_lib_state_machine.vi"("State(s) in Front (\"\")"="/* Post Error States", "State(s) in (\"\")"=w400) -> ("States Out"=w399:string)  [unwired: 13 in]
      }
      frame "Exit" {
        # "Do not put any code in this frame.\n(No errors that occur here will be handled.)"
        n188 = call <vilib>:"Add State(s) to Queue__jki_lib_state_machine.vi"("State(s) in (\"\")"=w405) -> ("States Out"=w404:string)  [unwired: 14 in]
      }
      frame "---------- Data ----------" {
        # "Do not put any code in this frame.\n(It is a separator no-op. You can make a copy of this frame to create a new Data frame)"
        n189 = call <vilib>:"Add State(s) to Queue__jki_lib_state_machine.vi"("State(s) in (\"\")"=w409) -> ("States Out"=w408:string)  [unwired: 14 in]
      }
      frame "Data: Initialize" {
        w410 = FALSE  # Fire Continues Allowed
        w412 = u32 0  # Tik1
        w411 = u32 0  # Tik2
        w413 = FALSE  # Jet trigger
        w414 = 0.0  # Discharge timing offset
        w415 = 0.0  # Heater timing offset
        w416 = T14 {"Current VI Reference"=refnum, "Close Panel on Exit?"=FALSE}  # Core
        # "Data names and types of shift register data are defined by this bundle."
        # "Initialize the shift-register data, here.\n(data names are defined by what you wire into the bundle function)"
        n190 = Bundle("Core"=w416, "Heater timing offset"=w415, "Discharge timing offset"=w414, "Jet trigger"=w413, "Tik1"=w412, "Tik2"=w411, "Fire Continues Allowed"=w410) -> (w418:T13)  [unwired: 1 in]
        n191 = call <vilib>:"Add State(s) to Queue__jki_lib_state_machine.vi"("State(s) in (\"\")"=w420) -> ("States Out"=w419:string)  [unwired: 14 in]
      }
      frame "Data: Cleanup" {
        # "Cleanup any data and references, here.\n(this is called automatically, by the Macro: Exit)"
        n192 = Unbundle By Name(w421) -> ("Core.Current VI Reference"=w424:refnum<vi>)
        n193 = Close Reference(reference=w424, error in (no error)=w423) -> (error out=w422:errorcluster)
        n194 = call <vilib>:"Add State(s) to Queue__jki_lib_state_machine.vi"("State(s) in (\"\")"=w426) -> ("States Out"=w425:string)  [unwired: 14 in]
      }
      frame "---------- UI ----------" {
        # "Do not put any code in this frame.\n(It is a separator no-op. You can make a copy of this frame to create a new UI frame)"
        n195 = call <vilib>:"Add State(s) to Queue__jki_lib_state_machine.vi"("State(s) in (\"\")"=w430) -> ("States Out"=w429:string)  [unwired: 14 in]
      }
      frame "UI: Initialize" {
        # "Initialize the User Interface, here.\n(this is called automatically, by the Macro: Init)"
        n196 = call <userlib>:"Fit VI window to Largest Dec__ogtk.vi"() -> ()  [unwired: 6 in, 2 out]
        n197 = call <vilib>:"Add State(s) to Queue__jki_lib_state_machine.vi"("State(s) in (\"\")"=w434) -> ("States Out"=w433:string)  [unwired: 14 in]
      }
      frame "UI: Cursor Set" {
        # "Argument"
        # "Set and Unset Cursor Busy.\n(Usage: \"UI: Cursor Set >> Busy|Idle\")"
        n198 = case shown="\"Idle\", Default" w435 {
          tunnel: w437 -> [w442 w444]
          tunnel: [w441 w443] -> w436
          frame "Idle", Default {
            n199 = call <vilib>:"Unset Busy.vi"("error in (no error)"=w442) -> ("error out"=w441:errorcluster)  [unwired: 10 in]
          }
          frame "Busy" {
            n200 = call <vilib>:"Set Busy.vi"("error in (no error)"=w444) -> ("error out"=w443:errorcluster)  [unwired: 9 in, 1 out]
          }
        }
        n201 = call <vilib>:"Add State(s) to Queue__jki_lib_state_machine.vi"("State(s) in (\"\")"=w440) -> ("States Out"=w439:string)  [unwired: 14 in]
      }
      frame "UI: Front Panel State" {
        # "Argument"
        # "Set Front Panel Open or Closed\n(Usage: \"UI: Front Panel State >> Open|Close\")"
        n202 = Unbundle By Name(w447) -> ("Core.Current VI Reference"=w446:refnum<vi>)
        n203 = case shown="\"Close\"" w445 {
          tunnel: w449 -> [w455 w468]
          tunnel: [w457 w469] -> w448
          tunnel: w446 -> [w456 w466]
          frame "Open", Default {
            n204 = property class="VI"(reference=w456, error in=w455) -> (reference out=w453:refnum<vi>, error out=w454:errorcluster, "Front Panel.Open"=w452:bool)
            n205 = case shown="False" w452 {
              tunnel: [w460 w463] -> w457
              tunnel: w454 -> [w459 w463]
              tunnel: w453 -> [w458 _]
              frame False {
                n206 = invoke class="VI" method="FP.Open"(reference=w458, error in=w459, "Activate"=TRUE, "State"=T9."Standard") -> (error out=w460:errorcluster)  [unwired: 1 in, 4 out]
              }
              frame True {
              }
            }
          }
          frame "Close" {
            n207 = property class="VI"(reference=w466, error in=w468) -> (reference out=w465:refnum<vi>, error out=w467:errorcluster, "Front Panel.Open"=w464:bool)
            n208 = case shown="True" w464 {
              tunnel: [w470 w473] -> w469
              tunnel: w467 -> [w470 w472]
              tunnel: w465 -> [_ w471]
              frame False {
              }
              frame True {
                n209 = invoke class="VI" method="FP.Close"(reference=w471, error in=w472) -> (error out=w473:errorcluster)  [unwired: 1 in, 2 out]
              }
            }
          }
        }
        n210 = call <vilib>:"Add State(s) to Queue__jki_lib_state_machine.vi"("State(s) in (\"\")"=w451) -> ("States Out"=w450:string)  [unwired: 14 in]
      }
      frame "---------- Macro ----------" {
        # "Do not put any code in this frame.\n(It is a separator no-op. You can make a copy of this frame to create a new Macro frame)"
        n211 = call <vilib>:"Add State(s) to Queue__jki_lib_state_machine.vi"("State(s) in (\"\")"=w477) -> ("States Out"=w476:string)  [unwired: 14 in]
      }
      frame "Macro: Initialize" {
        w478 = "Data: Initialize\nInitialize Core Data\nUI: Initialize\nUI: Front Panel State >> Open\nCheck if Fire continues allowed\nInitilize Fire Continues\nInit:MegattenuatorStage"  # Data: Initialize Initialize Core Data UI: Initialize UI: Front Panel State >> Open Check if Fire continues allowed Initilize Fire Continues Init:MegattenuatorStage
        # "Initialization Macro\n(This is called once, when the VI starts)"
        n212 = call <vilib>:"Add State(s) to Queue__jki_lib_state_machine.vi"("State(s) in Front (\"\")"=w478, "State(s) in (\"\")"=w482) -> ("States Out"=w481:string)  [unwired: 13 in]
      }
      frame "Macro: Exit" {
        # "Exit Macro\n(This is called once, when the VI exits)"
        n213 = Unbundle By Name(w492) -> ("Core.Close Panel on Exit?"=w491:bool)
        n214 = Release Queue(queue=w484, force destroy? (F)=TRUE) -> (error out=w483:errorcluster)  [unwired: 1 in, 2 out]
        n215 = call <vilib>:"Clear Errors.vi"("error in (no error)"=w483) -> ()  [unwired: 5 in, 2 out]
        n216 = Select(t="UI: Front Panel State >> Close", s=w491, f="") -> (s? t:f=w488:string)
        n217 = call <vilib>:"Add State(s) to Queue__jki_lib_state_machine.vi"("State(s) in (\"\")"=w488, "State(s) at Back (\"\")"="Data: Cleanup\nExit") -> ("States Out"=w486:string)  [unwired: 13 in]
        n218 = call <vilib>:"Add State(s) to Queue__jki_lib_state_machine.vi"("State(s) in Front (\"\")"=w486, "State(s) in (\"\")"=w495) -> ("States Out"=w494:string)  [unwired: 13 in]
      }
      frame "---------- New Category ----------" {
        # "Template Separator\n(You can make a copy of, or modify, this frame)"
        n219 = call <vilib>:"Add State(s) to Queue__jki_lib_state_machine.vi"("State(s) in (\"\")"=w499) -> ("States Out"=w498:string)  [unwired: 14 in]
      }
      frame "Check Megattenuator Stage Status" {
        n220 = property on="Position.Ch1::44" class="DigNum (strict)"() -> ("Value"=w500:dbl)  [unwired: 2 in, 2 out]
        n221 = case shown="2, Default" w500 {
          tunnel: ["IN" "Unknown/Moving" "OUT"] -> w501
          frame 0, 1 {
            n222 = property on="MoveStage" class="Bool (strict)"("Value"=TRUE) -> ()  [unwired: 2 in, 2 out]
          }
          frame 2, Default {
          }
          frame 149..151 {
            n223 = property on="MoveStage" class="Bool (strict)"("Value"=FALSE) -> ()  [unwired: 2 in, 2 out]
          }
        }
        n224 = property on="CurrentStatus" class="Str"("Value"=w501) -> ()  [unwired: 2 in, 2 out]
        n225 = call <vilib>:"Add State(s) to Queue__jki_lib_state_machine.vi"("State(s) in (\"\")"=w505) -> ("States Out"=w504:string)  [unwired: 14 in]
      }
      frame "Init:MegattenuatorStage" {
        # "Template Separator\n(You can make a copy of, or modify, this frame)"
        n226 = disable-structure shown="Disabled" {
          frame Disabled {
            n227 = flat-sequence {
              frame #0 {
                n228 = call <vilib>:"Set Busy.vi"("disable click? (T)"=TRUE, "cursor ID"=refnum<k1> refnum) -> ()  [unwired: 8 in, 2 out]
              }
              frame #1 {
                n229 = while {
                  tunnel: [w526] -> w518
                  i -> [w521]
                  stop <- w522 stop-if-true
                  n230 = Equal?(x=50, y=w521) -> (x = y?=w519:bool)
                  n231 = Not Equal?(x=w526, y=0.0) -> (x != y?=w523:bool)
                  n232 = Wait (ms)(milliseconds to wait=u32 100) -> ()  [unwired: 1 out]
                  n233 = Or(x=w523, y=w519) -> (x .or. y?=w522:bool)
                }
                n234 = case shown="0, 1" w518 {
                  tunnel: ["IN" "Unknown" "OUT"] -> w517
                  frame 0, 1 {
                    n235 = property on="MoveStage" class="Bool (strict)"("Value"=TRUE) -> ()  [unwired: 2 in, 2 out]
                  }
                  frame 2, Default {
                    n236 = property on="MoveStage" class="Bool (strict)"("DisabledEnum"=T7."Disabled" ("Disabled")) -> ()  [unwired: 2 in, 2 out]
                  }
                  frame 149..151 {
                    n237 = property on="MoveStage" class="Bool (strict)"("Value"=FALSE) -> ()  [unwired: 2 in, 2 out]
                  }
                }
                n238 = property on="CurrentStatus" class="Str"("Value"=w517) -> ()  [unwired: 2 in, 2 out]
              }
              frame #2 {
                n239 = call <vilib>:"Unset Busy.vi"() -> ()  [unwired: 11 in, 1 out]
              }
            }
          }
          frame Enabled {
          }
        }
        n240 = call <vilib>:"Add State(s) to Queue__jki_lib_state_machine.vi"("State(s) in (\"\")"=w514) -> ("States Out"=w513:string)  [unwired: 14 in]
      }
      frame "CheckTimeFire" {
        # "Your code here.\n(You can make a copy of, or modify, this frame)"
        n241 = Unbundle By Name(w539) -> ("Tik1"=w544:u32)
        n242 = Tick Count (ms)() -> (millisecond timer value=w546:u32)
        n243 = Unbundle By Name(w539) -> ("Fire Continues Allowed"=w536:bool)
        n244 = Reciprocal(x="Rate (Hz)") -> (1/x=w535:dbl)
        n245 = Subtract(x=w546, y=w544) -> (x-y=w547:u32)
        n246 = Multiply(x=1000.0, y=w535) -> (x*y=w534:dbl)
        n247 = Greater?(x=w547, y=w534) -> (0:w542:bool)
        n248 = And(x=w542, y="value0::22") -> (x .and. y?=w538:bool)
        n249 = And(x=w536, y=w538) -> (x .and. y?=w537:bool)
        n250 = case shown="True" w537 {
          tunnel: w546 -> [_ w554]
          tunnel: [w552 w554] -> w545
          tunnel: w544 -> [w552 _]
          tunnel: [_ "Action: Fire" ("State(s) in Front (\"\")")] -> w541
          frame False {
          }
          frame True {
          }
        }
        n251 = Bundle By Name(cluster=w539, "Tik1"=w545) -> (w548:T13)
        n252 = call <vilib>:"Add State(s) to Queue__jki_lib_state_machine.vi"("State(s) in Front (\"\")"=w541, "State(s) in (\"\")"=w551) -> ("States Out"=w550:string)  [unwired: 13 in]
        "Fire continues Indicator" <- "value0::22"
      }
      frame "Initilize Fire Continues" {
        # "Your code here.\n(You can make a copy of, or modify, this frame)"
        n253 = Unbundle By Name(w558) -> ("Fire Continues Allowed"=w557:bool)
        n254 = property on="value0::22" class="Bool (strict)"(error in=w560, "Visible"=w557) -> (error out=w559:errorcluster)  [unwired: 1 in, 1 out]
        n255 = Not(x=w557) -> (.not. x?=w555:bool)
        n256 = property on="Fire continues Indicator" class="Bool (strict)"(error in=w559, "Visible"=w555) -> (error out=w556:errorcluster)  [unwired: 1 in, 1 out]
        n257 = call <vilib>:"Add State(s) to Queue__jki_lib_state_machine.vi"("State(s) in (\"\")"=w562) -> ("States Out"=w561:string)  [unwired: 14 in]
      }
      frame "Check if Fire continues allowed" {
        # "Check if it is allowed computer"
        # "Your code here.\n(You can make a copy of, or modify, this frame)"
        n258 = String To IP() -> (0:w570:u32)  [unwired: 1 in]
        n259 = IP To String(1:TRUE ("dot notation? (F)"), 2:w570) -> (0:w571:string)
        n260 = Equal?(x=w571, y="192.168.14.2") -> (x = y?=w565:bool)
        n261 = Not(x=w565) -> (.not. x?=w566:bool)
        n262 = Bundle By Name(cluster=w568, "Fire Continues Allowed"=w565) -> (w567:T13)
        n263 = property on="Allow Fire Continues" class="Bool (strict)"(error in=w564, "Visible"=w566) -> (error out=w563:errorcluster)  [unwired: 1 in, 1 out]
        n264 = call <vilib>:"Add State(s) to Queue__jki_lib_state_machine.vi"("State(s) in (\"\")"=w574) -> ("States Out"=w573:string)  [unwired: 14 in]
      }
      frame "CheckTime2" {
        # "Your code here.\n(You can make a copy of, or modify, this frame)"
        n265 = Unbundle By Name(w583) -> ("Tik2"=w576:u32)
        n266 = Tick Count (ms)() -> (millisecond timer value=w578:u32)
        n267 = Subtract(x=w578, y=w576) -> (x-y=w581:u32)
        n268 = Greater?(x=w581, y=5000) -> (0:w579:bool)
        n269 = case shown="True" w579 {
          tunnel: w578 -> [_ w589]
          tunnel: [w587 w589] -> w577
          tunnel: w576 -> [w587 _]
          tunnel: [_ "Action: update expt vars\nAction: save screenshot"] -> w575
          frame False {
          }
          frame True {
          }
        }
        n270 = Bundle By Name(cluster=w583, "Tik2"=w577) -> (w582:T13)
        n271 = call <vilib>:"Add State(s) to Queue__jki_lib_state_machine.vi"("State(s) in Front (\"\")"=w575, "State(s) in (\"\")"=w586) -> ("States Out"=w585:string)  [unwired: 13 in]
      }
      frame "Action: Fire" {
        n272 = property on="fire::10" class="Str"(error in=w591, "Val(Sgnl)"="fire>>force" ("Value (Signaling)")) -> (error out=w590:errorcluster)  [unwired: 1 in, 1 out]
        n273 = call <vilib>:"Add State(s) to Queue__jki_lib_state_machine.vi"("State(s) in (\"\")"=w595) -> ("States Out"=w594:string)  [unwired: 14 in]
      }
      frame "Action: update expt vars" {
        # "Your code here.\n(You can make a copy of, or modify, this frame)"
        n274 = call <vilib>:"Add State(s) to Queue__jki_lib_state_machine.vi"("State(s) in (\"\")"=w599) -> ("States Out"=w598:string)  [unwired: 14 in]
      }
      frame "Action: SendScanParameters" {
        w601 = T10 {"Channel"="", "Scan Start"=0.0, "Scan End"=0.0} ("On Time cluster")
        # "Your code here.\n(You can make a copy of, or modify, this frame)"
        n275 = Select(t="value12::42", s="value1::43", f=0.0) -> (s? t:f=w612:dbl)
        n276 = Bundle By Name(cluster=w601, "Channel"="A", "Scan Start"="value14::42", "Scan End"="value15::42") -> (w626:T10)
        n277 = Select(t="value13::42", s="value1::43", f=0.0) -> (s? t:f=w616:dbl)
        n278 = Bundle By Name(cluster=T10 {"Channel"="", "Scan Start"=0.0, "Scan End"=0.0} ("On Time cluster"), "Channel"="B", "Scan Start"=w612, "Scan End"=w616) -> (w610:T10)
        n279 = Bundle By Name(cluster=w601, "Channel"="C", "Scan Start"=1.0, "Scan End"=0.0) -> (w622:T10)
        n280 = Bundle By Name(cluster=w601, "Channel"="E", "Scan Start"=1.0, "Scan End"=0.0) -> (w600:T10)
        n281 = Build Array(w626, w622, w600) -> (w621:T10[])
        n282 = Build Array(w610) -> (w608:T10[])
        n283 = call "BELLA PW scan mode shot control shutter.vi"("Expt editor SCS on"=w621, "PostScanRate"="value6::42", "ScanShotControl"="value0::43") -> ("error out"=w606:errorcluster, "delay F to set"=w629:dbl)  [unwired: 7 in]
        n284 = property on="Delay.Ch F::10" class="DigNum (strict)"("Val(Sgnl)"=w629) -> ()  [unwired: 2 in, 2 out]
        n285 = call "create and send sql query expt editor scan start end SRS delays.vi"("error in (no error)"=w606, "Array"=w608, "exptdeviceID"="840") -> ("error out"=w605:errorcluster)  [unwired: 8 in]
        n286 = disable-structure shown="Disabled" {
          frame Disabled {
            n287 = Select(f=0.0) -> ()  [unwired: 2 in, 1 out]
            n288 = Bundle By Name(cluster=T10 {"Channel"="", "Scan Start"=0.0, "Scan End"=0.0} ("On Time cluster"), "Channel"="A", "Scan Start"=1.045, "Scan End"=0.045) -> ()  [unwired: 1 out]
          }
          frame Enabled {
          }
        }
        n289 = flat-sequence {
          tunnel: w605 -> [_]
          frame #0 {
            n290 = call "TimeoutDialog.vi"("message 2"="expt editor set up" ("message"), "Timeout(ms)"=u32 1000) -> ()  [unwired: 9 in]
          }
        }
        n291 = disable-structure shown="Enabled" {
          disable-tunnel: _ -> [w641 _]
          disable-tunnel: _ -> [w640 _]
          frame Disabled {
            n292 = call "Jet in scan on or off.vi"("Jet On Times"=w641, "GasJetOn"=w640) -> ("error in (no error)"=w642:errorcluster)  [unwired: 8 in, 1 out]
          }
          frame Enabled {
          }
        }
        n293 = call <vilib>:"Add State(s) to Queue__jki_lib_state_machine.vi"("State(s) in (\"\")"=w634) -> ("States Out"=w633:string)  [unwired: 14 in]
      }
      frame "Action: save screenshot" {
        # "Your code here.\n(You can make a copy of, or modify, this frame)"
        n294 = case shown="True" "Save \ncreenshots" {
          frame False {
          }
          frame True {
            n295 = invoke class="VI" method="FP.Get Image"() -> ("image data"=w652:T11)  [unwired: 6 in, 5 out]
            n296 = call <vilib>:"Write PNG File.vi"("image data"=w652, "path to PNG file"=path "N:/data/ECS dumps/Logmaker Screenshot/frontpanel.png" ("report file path")) -> ("error out"=→"error out":errorcluster)  [unwired: 8 in, 1 out]
          }
        }
        n297 = call <vilib>:"Add State(s) to Queue__jki_lib_state_machine.vi"("State(s) in (\"\")"=w649) -> ("States Out"=w648:string)  [unwired: 14 in]
      }
    }
  }
  n298 = for {
    N: 25 -> [_]
    tunnel: w4 -> [w655]
    tunnel: [w655] -> w3
    tunnel: [w653] -> w1
    stop <- w653 stop-if-true
    n299 = local read "got manpar ofi data"() -> (w657:bool)
    n300 = local read "got manpar ofi bool data"() -> (w656:bool)
    n301 = Wait (ms)(milliseconds to wait=u32 1000) -> ()  [unwired: 1 out]
    n302 = And(x=w657, y=w656) -> (x .and. y?=w653:bool)
  }
  n303 = case shown="True" w1 {
    tunnel: w3 -> [_ w658]
    frame False {
    }
    frame True {
      n304 = call <userlib>:"Wait (ms)__ogtk.vi"("error in (no error)"=w658, "milliseconds to wait"=u32 3000) -> ("error out"=w660:errorcluster)  [unwired: 8 in, 1 out]
      n305 = property on="set expt editor" class="Bool (strict)"(error in=w660, "Val(Sgnl)"=TRUE ("Value (Signaling)")) -> ()  [unwired: 1 in, 2 out]
    }
  }
  "CurrentStatus" <- ""
